vi "220512-VNA RP FLAT.vi"() -> ()   [LabVIEW 2021]
uses:
  Channel parameters.ctl
  Spectrum data.ctl
  vna settings.ctl
  Resonnance detection.ctl
  <vilib>/Analysis/baseanly.llb/Mean (DBL).vi
  <vilib>/Utility/file.llb/Write Delimited Spreadsheet (DBL).vi
  <vilib>/regexp/Match Regular Expression.xnode
  <vilib>/Analysis/NI_AALBase.lvlib
panel:
  in  "Enable optical switch":bool
  in  "RP VNA SETTING":T1={"F start"=200000, "F stop"=2000500, "Sweep size"=1000, "Decimation"=5000, "F_corr"=0, "Ph_OUT1"=0, "Ph_OUT2"=0, "OUT_Lvl1"=32700, "OUT_Lvl2"=32700, "GPIO"=0}
  in  "Amplitude(1V)":dbl=0.3 format="%#_13g"
  out "RP CONNECT":bool
  in  "VOA Calibration cluster":cluster{"PUMP":dbl[], "PROBE":dbl[]}
  out "TRACK DATA REL NO SMOOTHING":dbl[][](array[numeric])
  out "TRACK DATA ABS NO SMOOTHING":dbl[][](array[numeric])
  in  "BTN SAVE TRACK":bool
  in  "BTN STOP TRACK":bool
  out "TRACK REPOSITERY":path
  out "TRACK DATA REL":dbl[][](array[numeric])
  out "TRACK DATA ABS":dbl[][](array[numeric])
  out "Track File List":path[](array[path])
  out "Track Repositery List":path[](array[path])
  out "CHANNEL CHOSEN":i32
  in  "TRACK-STOP":bool
  out "STATUS":string="STOP"
  out "track data":dbl[](array[numeric])=[495490.5081042979, 495481.56129759253, 495478.2328599854, 495479.84884744807, 495476.377462383, 495478.7819904735]
  out "MAIN TAB":T2(tab)
  in  "AVG Nb":i32=1 min=0 max=100 step=1
  in  "BTN AVG ENABLE":bool caption="AVERAGING"
  out "ACQ Indicator":bool
  in  "PUMP":dbl(slide)=100.0 min=0.0 max=100.0 step=0.1 scale=0.0..100.0
  in  "PROBE":dbl(slide)=100.0 min=0.0 max=100.0 step=0.1 scale=0.0..100.0
  in  "BTN RESET VNA":bool
  in  "SPAN":dbl=1900.0 format="%#5.1f"
  in  "STOP":dbl=2000.0 min=0.0 max=3000.0 format="%#5.1f"
  in  "CENTER":dbl=1050.0 format="%#5.1f"
  in  "BTN AF VNA":bool
  out "MAGNITUDE/PHASE":cluster{cluster{dbl, dbl}[]}[](graph)
  in  "CHANNEL CHOICE VNA":T3(radio)
  in  "BTN Center to max":bool
  in  "BTN ZOOM-":bool
  in  "BTN ZOOM+":bool
  in  "START":dbl=200.0 format="%#5.1f"
  out "SPACING":dbl=1900.0 min=0.0 max=100.0 step=0.5 format="%#5.1f"
  in  "Points N°":i32=1000 min=600 max=5000 step=1 format="%#4.4g"
  in  "BTN LOOP VNA":bool
  in  "BTN RUN VNA":bool
  in  "BTN SAVE VNA":bool
  in  "BTN FIT DISPLAY":bool caption="FIT DISPLAY"
  in  "BTN AUTOSCALE":bool=TRUE caption="AUTOSCALE"
  in  "BTN DISPLAY TYPE":bool caption="DISPLAY"
  in  "BTN VIEW PERSISTANCE":bool
  in  "BTN MAG/VEL":bool caption="DISPLAY"
  out "AVG Curr":i32=1 min=0 max=100 step=1
  in  "Hide/Show track data channel":bool[](array[boolean])
  in  "BTN AUTOSAVE RAW DATA":bool=TRUE
  in  "COMMENTS":string
  in  "ASSAY NAME":string
  in  "DELAY AFTER SWITCH (s)":i32
  in  "N°POINTS TO DISPLAY":i32=200
  in  "DISPLAY OPTION":u16(ring) items=["Absolute frequency", "Relative frequency (ppm)"]
  in  "DELAY BETWEEN TRIG (s)":i32
  in  "AVERAGE/POINT":dbl=1.0
  out "LIVE TRACK":dbl[][](graph)
  out "CHANNELS IND TRACK":T3(radio)
  in  "BTN RUN TRACK":bool
  in  "TEMPORAL SMOOTHING":i32=15
  in  "BTN NEW TRACK":bool
  in  "BTN PAUSE TRACK":bool
  in  "CHANNELS PARAMETERS":T4[](array[typedef])=[{"START 2"=200.0, "STOP 2"=2000.5, "CENTER 2"=1050.0, "SPAN 2"=1800.0, "CHANNEL TRACK ?"=FALSE, "PUMP"=100.0, "PROBE"=100.0, "Points N° 2"=1000, "SPACING 2"=100.0, "AVG"=0, "AVG ENABLE"=FALSE}, {"START 2"=200.0, "STOP 2"=2000.0, "CENTER 2"=1100.0, "SPAN 2"=1800.0, "CHANNEL TRACK ?"=FALSE, "PUMP"=100.0, "PROBE"=100.0, "Points N° 2"=1000, "SPACING 2"=1800.0, "AVG"=0, "AVG ENABLE"=FALSE}, {"START 2"=200.0, "STOP 2"=2000.0, "CENTER 2"=1100.0, "SPAN 2"=1800.0, "CHANNEL TRACK ?"=FALSE, "PUMP"=100.0, "PROBE"=100.0, "Points N° 2"=1000, "SPACING 2"=1800.0, "AVG"=0, "AVG ENABLE"=FALSE}, {"START 2"=200.0, "STOP 2"=2000.0, "CENTER 2"=1100.0, "SPAN 2"=1800.0, "CHANNEL TRACK ?"=FALSE, "PUMP"=100.0, "PROBE"=100.0, "Points N° 2"=1000, "SPACING 2"=1800.0, "AVG"=0, "AVG ENABLE"=FALSE}, {"START 2"=200.0, "STOP 2"=2000.0, "CENTER 2"=1100.0, "SPAN 2"=1800.0, "CHANNEL TRACK ?"=FALSE, "PUMP"=100.0, "PROBE"=100.0, "Points N° 2"=1000, "SPACING 2"=1800.0, "AVG"=0, "AVG ENABLE"=FALSE}, {"START 2"=200.0, "STOP 2"=2000.0, "CENTER 2"=1100.0, "SPAN 2"=1800.0, "CHANNEL TRACK ?"=FALSE, "PUMP"=100.0, "PROBE"=100.0, "Points N° 2"=1000, "SPACING 2"=1800.0, "AVG"=0, "AVG ENABLE"=FALSE}, {"START 2"=200.0, "STOP 2"=2000.0, "CENTER 2"=1100.0, "SPAN 2"=1800.0, "CHANNEL TRACK ?"=FALSE, "PUMP"=100.0, "PROBE"=100.0, "Points N° 2"=1000, "SPACING 2"=1800.0, "AVG"=0, "AVG ENABLE"=FALSE}, {"START 2"=200.0, "STOP 2"=2000.0, "CENTER 2"=1100.0, "SPAN 2"=1800.0, "CHANNEL TRACK ?"=FALSE, "PUMP"=100.0, "PROBE"=100.0, "Points N° 2"=1000, "SPACING 2"=1800.0, "AVG"=0, "AVG ENABLE"=FALSE}, {"START 2"=200.0, "STOP 2"=2000.0, "CENTER 2"=1100.0, "SPAN 2"=1800.0, "CHANNEL TRACK ?"=FALSE, "PUMP"=100.0, "PROBE"=100.0, "Points N° 2"=1000, "SPACING 2"=1800.0, "AVG"=0, "AVG ENABLE"=FALSE}, {"START 2"=200.0, "STOP 2"=2000.0, "CENTER 2"=1100.0, "SPAN 2"=1800.0, "CHANNEL TRACK ?"=FALSE, "PUMP"=100.0, "PROBE"=100.0, "Points N° 2"=1000, "SPACING 2"=1800.0, "AVG"=0, "AVG ENABLE"=FALSE}, {"START 2"=200.0, "STOP 2"=2000.0, "CENTER 2"=1100.0, "SPAN 2"=1800.0, "CHANNEL TRACK ?"=FALSE, "PUMP"=100.0, "PROBE"=100.0, "Points N° 2"=1000, "SPACING 2"=1800.0, "AVG"=0, "AVG ENABLE"=FALSE}, {"START 2"=200.0, "STOP 2"=2000.0, "CENTER 2"=1100.0, "SPAN 2"=1800.0, "CHANNEL TRACK ?"=FALSE, "PUMP"=100.0, "PROBE"=100.0, "Points N° 2"=1000, "SPACING 2"=1800.0, "AVG"=0, "AVG ENABLE"=FALSE}, {"START 2"=200.0, "STOP 2"=2000.0, "CENTER 2"=1100.0, "SPAN 2"=1800.0, "CHANNEL TRACK ?"=FALSE, "PUMP"=100.0, "PROBE"=100.0, "Points N° 2"=1000, "SPACING 2"=1800.0, "AVG"=0, "AVG ENABLE"=FALSE}, {"START 2"=200.0, "STOP 2"=2000.0, "CENTER 2"=1100.0, "SPAN 2"=1800.0, "CHANNEL TRACK ?"=FALSE, "PUMP"=100.0, "PROBE"=100.0, "Points N° 2"=1000, "SPACING 2"=1800.0, "AVG"=0, "AVG ENABLE"=FALSE}, {"START 2"=200.0, "STOP 2"=2000.0, "CENTER 2"=1100.0, "SPAN 2"=1800.0, "CHANNEL TRACK ?"=FALSE, "PUMP"=100.0, "PROBE"=100.0, "Points N° 2"=1000, "SPACING 2"=1800.0, "AVG"=0, "AVG ENABLE"=FALSE}, {"START 2"=200.0, "STOP 2"=2000.0, "CENTER 2"=1100.0, "SPAN 2"=1800.0, "CHANNEL TRACK ?"=FALSE, "PUMP"=100.0, "PROBE"=100.0, "Points N° 2"=1000, "SPACING 2"=1800.0, "AVG"=0, "AVG ENABLE"=FALSE}] {"AVG" min=0 max=100 step=1; "SPACING 2" min=0.0 max=100.0 step=0.5; "Points N° 2" min=0 max=100 step=1; "PROBE" min=0.0 max=100.0 step=0.5; "PUMP" min=0.0 max=100.0 step=0.5}
  out "CHANNEL IND SETTINGS":T5(radio)
  in  "RESONNANCE DETECTION":T6={"METHOD"=0, "Parabolic fit"={"Span type"=0, "Fit span"=100.0}} {"Parabolic fit"."Span type" items=["Points N°", "Frequency (Hz)", "Span %"]; "METHOD" items=["Maximum amplitude", "Max on parabolic fit"]}
  in  "TRACK DATA PARAMETERS":cluster{"MAIN FOLDER":path}={"MAIN FOLDER"=path "C:/SensWay Data"}
  in  "SPECTRUM POST PROCESSING PARAMETERS":cluster{"N° SMOOTHING POINTS":i32}={"N° SMOOTHING POINTS"=50}
  in  "AUTOFOCUS PARAMETERS":cluster{"ITERATIONS":i32}={"ITERATIONS"=5}
  in  "CHANNELS":T7
  in  "NETWORK PARAMETERS":T8={"RP-IP 1"="192.168.0.3", "RP-IP 2"="192.168.0.4", "RP-MAC 1"="", "RP-MAC 2"=""}
  in  "DARK SUB ?":bool
  in  "VNA DATA CLUSTER":T9 {"Time Stamp Indicator - Long" format="%<%.0X %x>T"}
  in  "TRACK DATA CLUSTER":cluster{"CHANNEL":dbl, "KPI 1 TRACK":ext[]}
  out "LOOP ACT":bool
  out "RAW Freq table":dbl[](array[numeric])=[200000.0, 201802.3023023023, 203604.6046046046, 205406.9069069069, 207209.20920920922, 209011.51151151152, 210813.81381381382, 212616.1161161161, 214418.4184184184, 216220.7207207207, 218023.02302302304, 219825.32532532534, 221627.62762762763, 223429.92992992993, 225232.23223223223, 227034.53453453453, 228836.83683683682, 230639.13913913915, 232441.44144144145, 234243.74374374375, 236046.04604604605, 237848.34834834834, 239650.65065065064, 241452.95295295294, 243255.25525525527, 245057.55755755756, 246859.85985985986, 248662.16216216216, 250464.46446446446, 252266.76676676676, 254069.06906906905, 255871.37137137138, 257673.67367367368, 259475.97597597598, 261278.27827827827, 263080.5805805806, 264882.8828828829, 266685.18518518517, 268487.4874874875, 270289.7897897898, 272092.0920920921, 273894.39439439436, 275696.6966966967, 277498.998998999, 279301.3013013013, 281103.6036036036, 282905.9059059059, 284708.2082082082, 286510.51051051053, 288312.8128128128, 290115.1151151151, 291917.4174174174, 293719.7197197197, 295522.02202202205, 297324.3243243243, 299126.6266266266, 300928.9289289289, 302731.23123123124, 304533.5335335335, 306335.83583583584, 308138.1381381381, 309940.44044044043, 311742.74274274276, 313545.04504504503, 315347.34734734736, 317149.6496496496, 318951.95195195195, 320754.2542542543, 322556.55655655655, 324358.8588588588, 326161.16116116114, 327963.4634634635, 329765.76576576574, 331568.06806806807, 333370.37037037034, 335172.67267267266, 336974.974974975, 338777.27727727726, 340579.5795795796, 342381.88188188185, 344184.1841841842, 345986.4864864865, 347788.7887887888, 349591.09109109105, 351393.3933933934, 353195.6956956957, 354997.997997998, 356800.3003003003, 358602.60260260256, 360404.9049049049, 362207.2072072072, 364009.50950950955, 365811.8118118118, 367614.1141141141, 369416.4164164164, 371218.71871871874, 373021.021021021, 374823.3233233233, 376625.6256256256, 378427.9279279279, 380230.23023023026, 382032.5325325325, 383834.8348348348, 385637.1371371371, 387439.43943943945, 389241.7417417418, 391044.04404404404, 392846.3463463463, 394648.64864864864, 396450.95095095097, 398253.25325325324, 400055.5555555555, 401857.85785785783, 403660.16016016016, 405462.4624624625, 407264.76476476475, 409067.067067067, 410869.36936936935, 412671.6716716717, 414473.973973974, 416276.2762762763, 418078.57857857854, 419880.88088088087, 421683.1831831832, 423485.48548548546, 425287.7877877878, 427090.09009009006, 428892.3923923924, 430694.6946946947, 432496.996996997, 434299.29929929925, 436101.6016016016, 437903.9039039039, 439706.20620620623, 441508.5085085085, 443310.81081081077, 445113.1131131131, 446915.4154154154, 448717.7177177177, 450520.02002002, 452322.3223223223, 454124.6246246246, 455926.92692692694, 457729.2292292292, 459531.5315315315, 461333.8338338338, 463136.13613613613, 464938.4384384384, 466740.74074074073, 468543.04304304306, 470345.3453453453, 472147.64764764765, 473949.9499499499, 475752.25225225225, 477554.5545545545, 479356.85685685684, 481159.1591591592, 482961.46146146144, 484763.76376376377, 486566.06606606604, 488368.36836836836, 490170.67067067063, 491972.97297297296, 493775.2752752753, 495577.57757757755, 497379.8798798799, 499182.18218218215, 500984.4844844845, 502786.78678678675, 504589.0890890891, 506391.3913913914, 508193.69369369367, 509995.995995996, 511798.29829829826, 513600.6006006006, 515402.90290290286, 517205.2052052052, 519007.5075075075, 520809.8098098098, 522612.1121121121, 524414.4144144144, 526216.7167167168, 528019.0190190191, 529821.3213213213, 531623.6236236236, 533425.9259259258, 535228.2282282282, 537030.5305305305, 538832.8328328328, 540635.1351351351, 542437.4374374375, 544239.7397397398, 546042.042042042, 547844.3443443443, 549646.6466466465, 551448.9489489489, 553251.2512512512, 555053.5535535535, 556855.8558558559, 558658.1581581582, 560460.4604604605, 562262.7627627627, 564065.065065065, 565867.3673673674, 567669.6696696696, 569471.9719719719, 571274.2742742742, 573076.5765765766, 574878.8788788789, 576681.1811811812, 578483.4834834835, 580285.7857857858, 582088.0880880881, 583890.3903903903, 585692.6926926926, 587494.994994995, 589297.2972972973, 591099.5995995996, 592901.9019019019, 594704.2042042043, 596506.5065065065, 598308.8088088088, 600111.111111111, 601913.4134134133, 603715.7157157157, 605518.018018018, 607320.3203203203, 609122.6226226226, 610924.924924925, 612727.2272272272, 614529.5295295295, 616331.8318318318, 618134.134134134, 619936.4364364364, 621738.7387387387, 623541.041041041, 625343.3433433434, 627145.6456456457, 628947.947947948, 630750.2502502502, 632552.5525525525, 634354.8548548548, 636157.1571571571, 637959.4594594594, 639761.7617617617, 641564.0640640641, 643366.3663663664, 645168.6686686687, 646970.9709709709, 648773.2732732733, 650575.5755755756, 652377.8778778778, 654180.1801801801, 655982.4824824824, 657784.7847847848, 659587.0870870871, 661389.3893893894, 663191.6916916918, 664993.993993994, 666796.2962962963, 668598.5985985985, 670400.9009009008, 672203.2032032032, 674005.5055055055, 675807.8078078078, 677610.1101101101, 679412.4124124125, 681214.7147147147, 683017.017017017, 684819.3193193192, 686621.6216216215, 688423.9239239239, 690226.2262262262, 692028.5285285285, 693830.8308308308, 695633.1331331332, 697435.4354354354, 699237.7377377377, 701040.04004004, 702842.3423423423, 704644.6446446446, 706446.9469469469, 708249.2492492492, 710051.5515515516, 711853.8538538539, 713656.1561561562, 715458.4584584584, 717260.7607607607, 719063.063063063, 720865.3653653653, 722667.6676676676, 724469.9699699699, 726272.2722722723, 728074.5745745746, 729876.8768768768, 731679.1791791791, 733481.4814814815, 735283.7837837838, 737086.0860860861, 738888.3883883883, 740690.6906906907, 742492.992992993, 744295.2952952953, 746097.5975975975, 747899.8998998998, 749702.2022022022, 751504.5045045045, 753306.8068068068, 755109.109109109, 756911.4114114114, 758713.7137137137, 760516.016016016, 762318.3183183183, 764120.6206206206, 765922.9229229229, 767725.2252252252, 769527.5275275275, 771329.8298298299, 773132.1321321321, 774934.4344344344, 776736.7367367367, 778539.039039039, 780341.3413413413, 782143.6436436436, 783945.9459459459, 785748.2482482482, 787550.5505505506, 789352.8528528528, 791155.1551551551, 792957.4574574574, 794759.7597597598, 796562.0620620621, 798364.3643643643, 800166.6666666666, 801968.968968969, 803771.2712712713, 805573.5735735735, 807375.8758758758, 809178.1781781781, 810980.4804804805, 812782.7827827828, 814585.085085085, 816387.3873873873, 818189.6896896897, 819991.991991992, 821794.2942942943, 823596.5965965965, 825398.8988988989, 827201.2012012012, 829003.5035035035, 830805.8058058057, 832608.108108108, 834410.4104104104, 836212.7127127127, 838015.015015015, 839817.3173173172, 841619.6196196196, 843421.9219219219, 845224.2242242242, 847026.5265265265, 848828.8288288288, 850631.1311311311, 852433.4334334334, 854235.7357357357, 856038.0380380381, 857840.3403403403, 859642.6426426426, 861444.9449449449, 863247.2472472473, 865049.5495495495, 866851.8518518518, 868654.1541541541, 870456.4564564564, 872258.7587587588, 874061.061061061, 875863.3633633633, 877665.6656656656, 879467.967967968, 881270.2702702703, 883072.5725725725, 884874.8748748748, 886677.1771771772, 888479.4794794795, 890281.7817817817, 892084.084084084, 893886.3863863864, 895688.6886886887, 897490.990990991, 899293.2932932932, 901095.5955955955, 902897.8978978979, 904700.2002002002, 906502.5025025025, 908304.8048048047, 910107.1071071071, 911909.4094094094, 913711.7117117117, 915514.0140140139, 917316.3163163163, 919118.6186186186, 920920.9209209209, 922723.2232232232, 924525.5255255254, 926327.8278278278, 928130.1301301301, 929932.4324324324, 931734.7347347348, 933537.037037037, 935339.3393393393, 937141.6416416416, 938943.943943944, 940746.2462462463, 942548.5485485485, 944350.8508508508, 946153.1531531531, 947955.4554554555, 949757.7577577577, 951560.06006006, 953362.3623623623, 955164.6646646647, 956966.966966967, 958769.2692692692, 960571.5715715715, 962373.8738738738, 964176.1761761762, 965978.4784784785, 967780.7807807807, 969583.083083083, 971385.3853853854, 973187.6876876877, 974989.9899899899, 976792.2922922922, 978594.5945945946, 980396.8968968969, 982199.1991991992, 984001.5015015014, 985803.8038038037, 987606.1061061061, 989408.4084084084, 991210.7107107107, 993013.0130130129, 994815.3153153153, 996617.6176176176, 998419.9199199199, 1000222.2222222221, 1002024.5245245245, 1003826.8268268268, 1005629.1291291291, 1007431.4314314314, 1009233.7337337337, 1011036.036036036, 1012838.3383383383, 1014640.6406406406, 1016442.942942943, 1018245.2452452452, 1020047.5475475475, 1021849.8498498498, 1023652.1521521521, 1025454.4544544544, 1027256.7567567567, 1029059.059059059, 1030861.3613613613, 1032663.6636636637, 1034465.9659659659, 1036268.2682682682, 1038070.5705705705, 1039872.8728728729, 1041675.1751751752, 1043477.4774774774, 1045279.7797797797, 1047082.082082082, 1048884.3843843844, 1050686.6866866867, 1052488.988988989, 1054291.2912912914, 1056093.5935935937, 1057895.895895896, 1059698.198198198, 1061500.5005005004, 1063302.8028028028, 1065105.105105105, 1066907.4074074074, 1068709.7097097095, 1070512.0120120118, 1072314.3143143142, 1074116.6166166165, 1075918.9189189188, 1077721.2212212211, 1079523.5235235235, 1081325.8258258258, 1083128.1281281281, 1084930.4304304305, 1086732.7327327328, 1088535.035035035, 1090337.3373373374, 1092139.6396396398, 1093941.9419419419, 1095744.2442442442, 1097546.5465465465, 1099348.8488488488, 1101151.1511511512, 1102953.4534534533, 1104755.7557557556, 1106558.058058058, 1108360.3603603602, 1110162.6626626626, 1111964.964964965, 1113767.2672672672, 1115569.5695695695, 1117371.8718718719, 1119174.1741741742, 1120976.4764764765, 1122778.7787787789, 1124581.0810810812, 1126383.3833833835, 1128185.6856856856, 1129987.987987988, 1131790.2902902903, 1133592.5925925926, 1135394.894894895, 1137197.197197197, 1138999.4994994993, 1140801.8018018017, 1142604.104104104, 1144406.4064064063, 1146208.7087087086, 1148011.011011011, 1149813.3133133133, 1151615.6156156156, 1153417.917917918, 1155220.2202202203, 1157022.5225225226, 1158824.824824825, 1160627.1271271273, 1162429.4294294294, 1164231.7317317317, 1166034.034034034, 1167836.3363363363, 1169638.6386386384, 1171440.9409409408, 1173243.243243243, 1175045.5455455454, 1176847.8478478477, 1178650.15015015, 1180452.4524524524, 1182254.7547547547, 1184057.057057057, 1185859.3593593594, 1187661.6616616617, 1189463.963963964, 1191266.2662662663, 1193068.5685685687, 1194870.8708708708, 1196673.173173173, 1198475.4754754754, 1200277.7777777778, 1202080.08008008, 1203882.3823823822, 1205684.6846846845, 1207486.9869869868, 1209289.2892892892, 1211091.5915915915, 1212893.8938938938, 1214696.1961961961, 1216498.4984984985, 1218300.8008008008, 1220103.103103103, 1221905.4054054054, 1223707.7077077078, 1225510.01001001, 1227312.3123123124, 1229114.6146146145, 1230916.9169169168, 1232719.2192192192, 1234521.5215215215, 1236323.8238238238, 1238126.126126126, 1239928.4284284282, 1241730.7307307306, 1243533.033033033, 1245335.3353353352, 1247137.6376376376, 1248939.9399399399, 1250742.2422422422, 1252544.5445445445, 1254346.8468468469, 1256149.1491491492, 1257951.4514514515, 1259753.7537537536, 1261556.056056056, 1263358.3583583583, 1265160.6606606606, 1266962.962962963, 1268765.2652652652, 1270567.5675675676, 1272369.86986987, 1274172.1721721722, 1275974.4744744743, 1277776.7767767766, 1279579.079079079, 1281381.3813813813, 1283183.6836836836, 1284985.985985986, 1286788.2882882883, 1288590.5905905906, 1290392.892892893, 1292195.195195195, 1293997.4974974974, 1295799.7997997997, 1297602.102102102, 1299404.4044044043, 1301206.7067067067, 1303009.009009009, 1304811.3113113113, 1306613.6136136136, 1308415.915915916, 1310218.218218218, 1312020.5205205204, 1313822.8228228227, 1315625.125125125, 1317427.4274274274, 1319229.7297297297, 1321032.032032032, 1322834.3343343344, 1324636.6366366367, 1326438.9389389388, 1328241.241241241, 1330043.5435435434, 1331845.8458458458, 1333648.148148148, 1335450.4504504504, 1337252.7527527527, 1339055.055055055, 1340857.3573573574, 1342659.6596596597, 1344461.9619619618, 1346264.2642642641, 1348066.5665665665, 1349868.8688688688, 1351671.1711711711, 1353473.4734734735, 1355275.7757757758, 1357078.078078078, 1358880.3803803804, 1360682.6826826825, 1362484.9849849849, 1364287.2872872872, 1366089.5895895895, 1367891.8918918918, 1369694.1941941942, 1371496.4964964965, 1373298.7987987988, 1375101.1011011011, 1376903.4034034032, 1378705.7057057056, 1380508.008008008, 1382310.3103103102, 1384112.6126126125, 1385914.9149149149, 1387717.2172172172, 1389519.5195195195, 1391321.8218218219, 1393124.1241241242, 1394926.4264264263, 1396728.7287287286, 1398531.031031031, 1400333.3333333333, 1402135.6356356356, 1403937.937937938, 1405740.2402402402, 1407542.5425425426, 1409344.844844845, 1411147.147147147, 1412949.4494494493, 1414751.7517517516, 1416554.054054054, 1418356.3563563563, 1420158.6586586586, 1421960.960960961, 1423763.2632632633, 1425565.5655655656, 1427367.867867868, 1429170.17017017, 1430972.4724724723, 1432774.7747747747, 1434577.077077077, 1436379.3793793793, 1438181.6816816817, 1439983.983983984, 1441786.2862862863, 1443588.5885885886, 1445390.8908908907, 1447193.193193193, 1448995.4954954954, 1450797.7977977977, 1452600.1001001, 1454402.4024024024, 1456204.7047047047, 1458007.007007007, 1459809.3093093093, 1461611.6116116114, 1463413.9139139138, 1465216.216216216, 1467018.5185185184, 1468820.8208208208, 1470623.123123123, 1472425.4254254254, 1474227.7277277277, 1476030.03003003, 1477832.3323323324, 1479634.6346346345, 1481436.9369369368, 1483239.2392392391, 1485041.5415415415, 1486843.8438438438, 1488646.146146146, 1490448.4484484484, 1492250.7507507508, 1494053.053053053, 1495855.3553553552, 1497657.6576576575, 1499459.9599599598, 1501262.2622622622, 1503064.5645645645, 1504866.8668668668, 1506669.1691691692, 1508471.4714714715, 1510273.7737737738, 1512076.0760760761, 1513878.3783783782, 1515680.6806806806, 1517482.9829829829, 1519285.2852852852, 1521087.5875875875, 1522889.8898898899, 1524692.1921921922, 1526494.4944944945, 1528296.7967967968, 1530099.099099099, 1531901.4014014013, 1533703.7037037036, 1535506.006006006, 1537308.3083083082, 1539110.6106106106, 1540912.912912913, 1542715.2152152152, 1544517.5175175176, 1546319.8198198196, 1548122.122122122, 1549924.4244244243, 1551726.7267267266, 1553529.029029029, 1555331.3313313313, 1557133.6336336336, 1558935.935935936, 1560738.2382382383, 1562540.5405405406, 1564342.8428428427, 1566145.145145145, 1567947.4474474473, 1569749.7497497497, 1571552.052052052, 1573354.3543543543, 1575156.6566566566, 1576958.958958959, 1578761.2612612613, 1580563.5635635634, 1582365.8658658657, 1584168.168168168, 1585970.4704704704, 1587772.7727727727, 1589575.075075075, 1591377.3773773774, 1593179.6796796797, 1594981.981981982, 1596784.2842842843, 1598586.5865865864, 1600388.8888888888, 1602191.191191191, 1603993.4934934934, 1605795.7957957957, 1607598.098098098, 1609400.4004004004, 1611202.7027027027, 1613005.005005005, 1614807.3073073071, 1616609.6096096095, 1618411.9119119118, 1620214.2142142141, 1622016.5165165165, 1623818.8188188188, 1625621.121121121, 1627423.4234234234, 1629225.7257257258, 1631028.0280280279, 1632830.3303303302, 1634632.6326326325, 1636434.9349349348, 1638237.2372372372, 1640039.5395395395, 1641841.8418418418, 1643644.1441441441, 1645446.4464464465, 1647248.7487487488, 1649051.051051051, 1650853.3533533532, 1652655.6556556555, 1654457.9579579579, 1656260.2602602602, 1658062.5625625625, 1659864.8648648649, 1661667.1671671672, 1663469.4694694695, 1665271.7717717716, 1667074.074074074, 1668876.3763763763, 1670678.6786786786, 1672480.980980981, 1674283.2832832832, 1676085.5855855856, 1677887.887887888, 1679690.1901901902, 1681492.4924924925, 1683294.7947947946, 1685097.097097097, 1686899.3993993993, 1688701.7017017016, 1690504.004004004, 1692306.3063063063, 1694108.6086086086, 1695910.910910911, 1697713.2132132133, 1699515.5155155153, 1701317.8178178177, 1703120.12012012, 1704922.4224224223, 1706724.7247247247, 1708527.027027027, 1710329.3293293293, 1712131.6316316316, 1713933.933933934, 1715736.236236236, 1717538.5385385384, 1719340.8408408407, 1721143.143143143, 1722945.4454454454, 1724747.7477477477, 1726550.05005005, 1728352.3523523523, 1730154.6546546547, 1731956.956956957, 1733759.259259259, 1735561.5615615614, 1737363.8638638637, 1739166.166166166, 1740968.4684684684, 1742770.7707707707, 1744573.073073073, 1746375.3753753754, 1748177.6776776777, 1749979.9799799798, 1751782.2822822821, 1753584.5845845845, 1755386.8868868868, 1757189.189189189, 1758991.4914914914, 1760793.7937937938, 1762596.096096096, 1764398.3983983984, 1766200.7007007005, 1768003.0030030028, 1769805.3053053052, 1771607.6076076075, 1773409.9099099098, 1775212.2122122122, 1777014.5145145145, 1778816.8168168168, 1780619.1191191191, 1782421.4214214215, 1784223.7237237236, 1786026.0260260259, 1787828.3283283282, 1789630.6306306305, 1791432.9329329329, 1793235.2352352352, 1795037.5375375375, 1796839.8398398398, 1798642.1421421422, 1800444.4444444443, 1802246.7467467466, 1804049.049049049, 1805851.3513513512, 1807653.6536536536, 1809455.955955956, 1811258.2582582582, 1813060.5605605606, 1814862.8628628629, 1816665.1651651652, 1818467.4674674673, 1820269.7697697696, 1822072.072072072, 1823874.3743743743, 1825676.6766766766, 1827478.978978979, 1829281.2812812813, 1831083.5835835836, 1832885.885885886, 1834688.188188188, 1836490.4904904903, 1838292.7927927927, 1840095.095095095, 1841897.3973973973, 1843699.6996996996, 1845502.002002002, 1847304.3043043043, 1849106.6066066066, 1850908.9089089087, 1852711.211211211, 1854513.5135135134, 1856315.8158158157, 1858118.118118118, 1859920.4204204204, 1861722.7227227227, 1863525.025025025, 1865327.3273273273, 1867129.6296296297, 1868931.9319319318, 1870734.234234234, 1872536.5365365364, 1874338.8388388387, 1876141.141141141, 1877943.4434434434, 1879745.7457457457, 1881548.048048048, 1883350.3503503504, 1885152.6526526525, 1886954.9549549548, 1888757.2572572571, 1890559.5595595594, 1892361.8618618618, 1894164.164164164, 1895966.4664664664, 1897768.7687687688, 1899571.071071071, 1901373.3733733734, 1903175.6756756755, 1904977.9779779778, 1906780.2802802802, 1908582.5825825825, 1910384.8848848848, 1912187.1871871871, 1913989.4894894895, 1915791.7917917918, 1917594.0940940941, 1919396.3963963962, 1921198.6986986985, 1923001.0010010009, 1924803.3033033032, 1926605.6056056055, 1928407.9079079079, 1930210.2102102102, 1932012.5125125125, 1933814.8148148148, 1935617.117117117, 1937419.4194194193, 1939221.7217217216, 1941024.024024024, 1942826.3263263262, 1944628.6286286286, 1946430.930930931, 1948233.2332332332, 1950035.5355355355, 1951837.8378378379, 1953640.14014014, 1955442.4424424423, 1957244.7447447446, 1959047.047047047, 1960849.3493493493, 1962651.6516516516, 1964453.953953954, 1966256.2562562563, 1968058.5585585586, 1969860.8608608607, 1971663.163163163, 1973465.4654654653, 1975267.7677677677, 1977070.07007007, 1978872.3723723723, 1980674.6746746746, 1982476.976976977, 1984279.2792792793, 1986081.5815815816, 1987883.8838838837, 1989686.186186186, 1991488.4884884884, 1993290.7907907907, 1995093.093093093, 1996895.3953953953, 1998697.6976976977, 2000500.0]
  in  "ENABLE INTERNAL MODULATION":bool=TRUE
  in  "VNA DATA CLUSTER TBL":T9[](array[typedef]) {"Time Stamp Indicator - Long" format="%<%.0X %x>T"}
  in  "TRACK DATA CLUSTER TBL":cluster{"CHANNEL":dbl, "KPI 1 TRACK":ext[]}[](array[cluster])=[{"CHANNEL"=0.0, "KPI 1 TRACK"=[]}, {"CHANNEL"=0.0, "KPI 1 TRACK"=[]}, {"CHANNEL"=0.0, "KPI 1 TRACK"=[]}, {"CHANNEL"=0.0, "KPI 1 TRACK"=[]}, {"CHANNEL"=0.0, "KPI 1 TRACK"=[]}, {"CHANNEL"=0.0, "KPI 1 TRACK"=[]}, {"CHANNEL"=0.0, "KPI 1 TRACK"=[]}, {"CHANNEL"=0.0, "KPI 1 TRACK"=[]}, {"CHANNEL"=0.0, "KPI 1 TRACK"=[]}, {"CHANNEL"=0.0, "KPI 1 TRACK"=[]}, {"CHANNEL"=0.0, "KPI 1 TRACK"=[]}, {"CHANNEL"=0.0, "KPI 1 TRACK"=[]}, {"CHANNEL"=0.0, "KPI 1 TRACK"=[]}, {"CHANNEL"=0.0, "KPI 1 TRACK"=[]}, {"CHANNEL"=0.0, "KPI 1 TRACK"=[]}, {"CHANNEL"=0.0, "KPI 1 TRACK"=[]}]
  in  "PERSISTANCE DATA CLUSTER":T9 {"Time Stamp Indicator - Long" format="%<%.0X %x>T"}
  in  "VNA SETTING CLUSTER":T4 {"AVG" min=0 max=100 step=1; "SPACING 2" min=0.0 max=100.0 step=0.5; "Points N° 2" min=0 max=100 step=1; "PROBE" min=0.0 max=100.0 step=0.5; "PUMP" min=0.0 max=100.0 step=0.5}
  out "Information tips":string
  in  "PANEL VNA":bool
  in  "PANEL TRACKING":bool
  in  "BTN STOP":bool
  in  "PANEL GENERAL SETTINGS":bool
  in  "PANEL TRACK SETTINGS":bool
  # "POINTS"
  # "SPACING"
  # "TRACK ?"
  # "START"
  # "STOP"
  # "CENTER"
  # "SPAN"
  # "PROBE"
  # "PUMP"
  # "AVERAGING"
  # "BETA ONLY !!!"
  # "PARAMETERS"
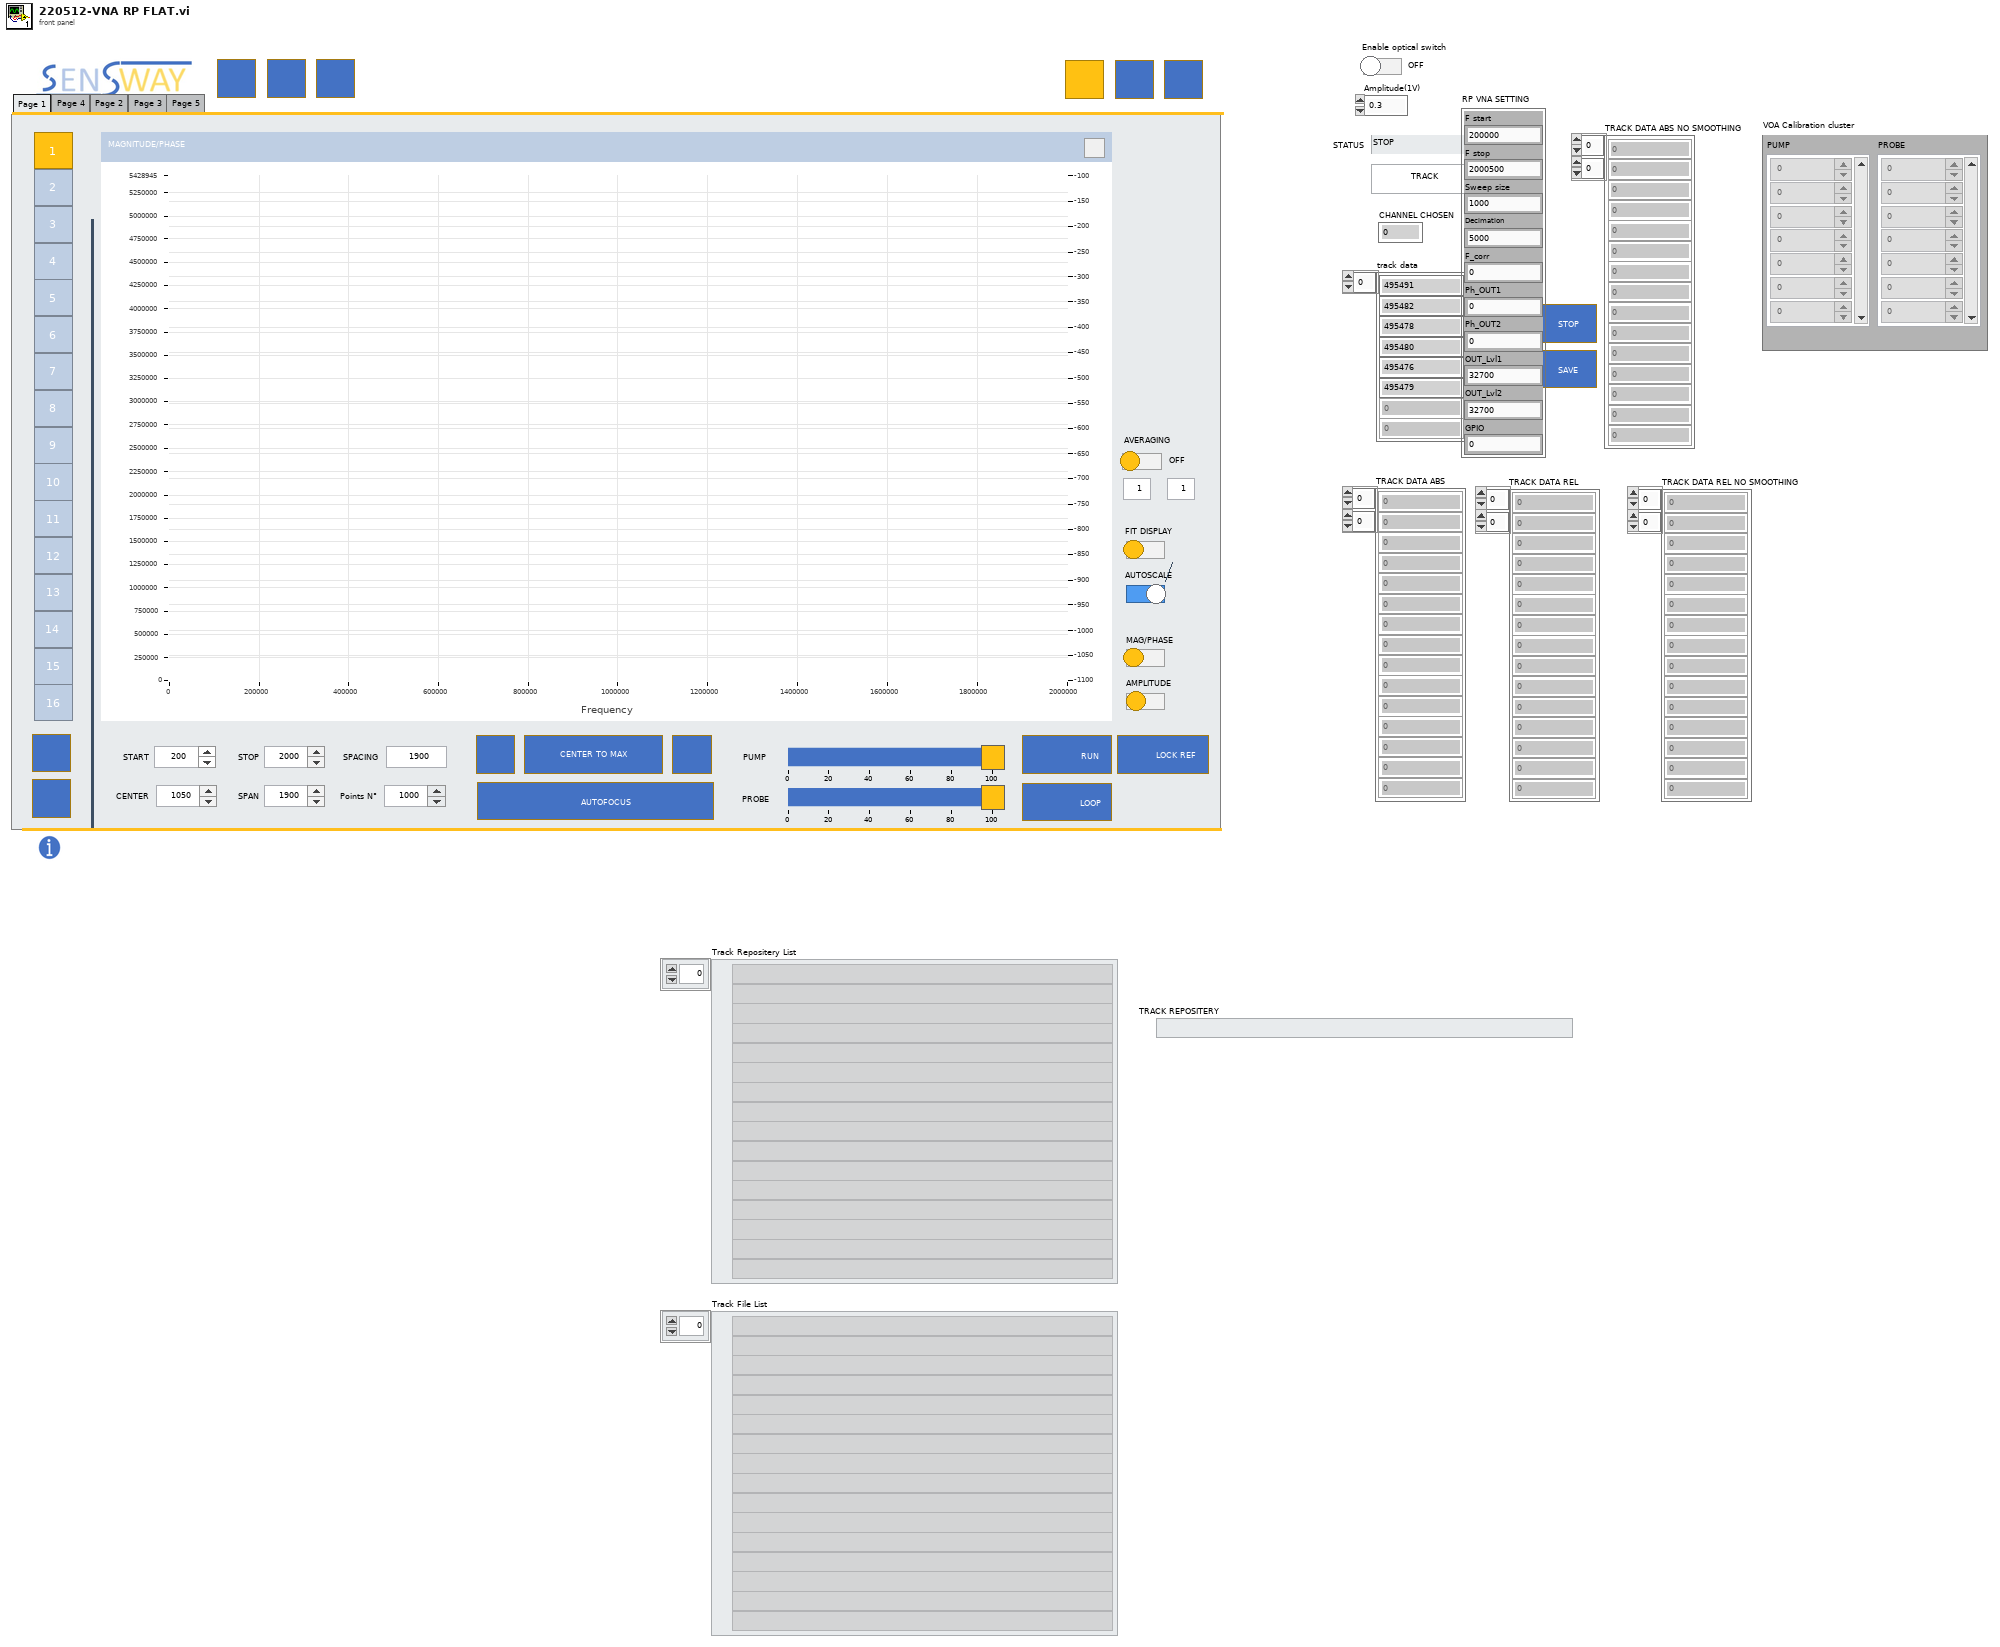
[diagram p1: front panel]
types:
  T1 = typedef "vna settings.ctl" = cluster{"F start":u32, "F stop":u32, "Sweep size":u32, "Decimation":u32, "F_corr":u32, "Ph_OUT1":u32, "Ph_OUT2":u32, "OUT_Lvl1":u32, "OUT_Lvl2":u32, "GPIO":u32}
  T2 = enum32{"Page 1", "Page 4", "Page 2", "Page 3", "Page 5"}
  T3 = enum32{"Button 1", "Button 2", "Button 3", "Sélection radio 4", "Sélection radio 5", "Sélection radio 6", "Sélection radio 7", "Sélection radio 8", "Sélection radio 9", "Sélection radio 10", "Sélection radio 11", "Sélection radio 12", "Sélection radio 13", "Sélection radio 14", "Sélection radio 15", "Sélection radio 16"}
  T4 = typedef "Channel parameters.ctl" = cluster{"START 2":dbl, "STOP 2":dbl, "CENTER 2":dbl, "SPAN 2":dbl, "CHANNEL TRACK ?":bool, "PUMP":dbl, "PROBE":dbl, "Points N° 2":i32, "SPACING 2":dbl, "AVG":i32, "AVG ENABLE":bool}
  T5 = enum32{"No Selection", "Button 1", "Button 2", "Button 3", "Sélection radio 4", "Sélection radio 5", "Sélection radio 6", "Sélection radio 7", "Sélection radio 8", "Sélection radio 9", "Sélection radio 10", "Sélection radio 11", "Sélection radio 12", "Sélection radio 13", "Sélection radio 14", "Sélection radio 15", "Sélection radio 16"}
  T6 = typedef "Resonnance detection.ctl" = cluster{"METHOD":u16, "Parabolic fit":cluster{"Span type":u16, "Fit span":dbl}}
  T7 = cluster{"CHANNEL 1":bool, "CHANNEL 2":bool, "CHANNEL 3":bool, "CHANNEL 4":bool, "CHANNEL 5":bool, "CHANNEL 6":bool, "CHANNEL 7":bool, "CHANNEL 8":bool, "CHANNEL 9":bool, "CHANNEL 10":bool, "CHANNEL 11":bool, "CHANNEL 12":bool, "CHANNEL 13":bool, "CHANNEL 14":bool, "CHANNEL 15":bool, "CHANNEL 16":bool}
  T8 = cluster{"RP-IP 1":string, "RP-IP 2":string, "RP-MAC 1":string, "RP-MAC 2":string}
  T9 = typedef "Spectrum data.ctl" = cluster{"CHANNEL":dbl, "FREQUENCY TABLE":ext[], "MAGNITUDE TABLE":ext[], "PHASE TABLE":ext[], "REAL TABLE":ext[], "IMAGINARY TABLE":ext[], "Time Stamp Indicator - Long":timestamp}
  T10 = enum16{"Freq start", "Freq stop", "Sweep size", "Decimation rate", "Freq corr", "Phase output 1", "Phase output 2", "Output level 1", "Output level 2", "GPIO", "SWEEP START"}
  T11 = enum8{"Enabled", "Disabled", "Disabled and Grayed Out"}
  T12 = cluster{"FREQUENCY":sgl[], "REAL 1":dbl[], "IMAGINARY 1":sgl[], "MAGNITUDE 1":dbl[], "PHASE 1":dbl[], "REAL 2":dbl[], "IMAGINARY 2":sgl[], "MAGNITUDE 2":dbl[], "PHASE 2":dbl[]}
  T13 = cluster{cluster{"Numeric Control":ext, "Numeric Control":ext}[]}[]
  T14 = cluster{"F start":u32, "F stop":u32, "Sweep size":u32, "Decimation":u32, "F_corr":u32, "Ph_OUT1":u32, "Ph_OUT2":u32, "OUT_Lvl1":u32, "OUT_Lvl2":u32, "GPIO":u32}
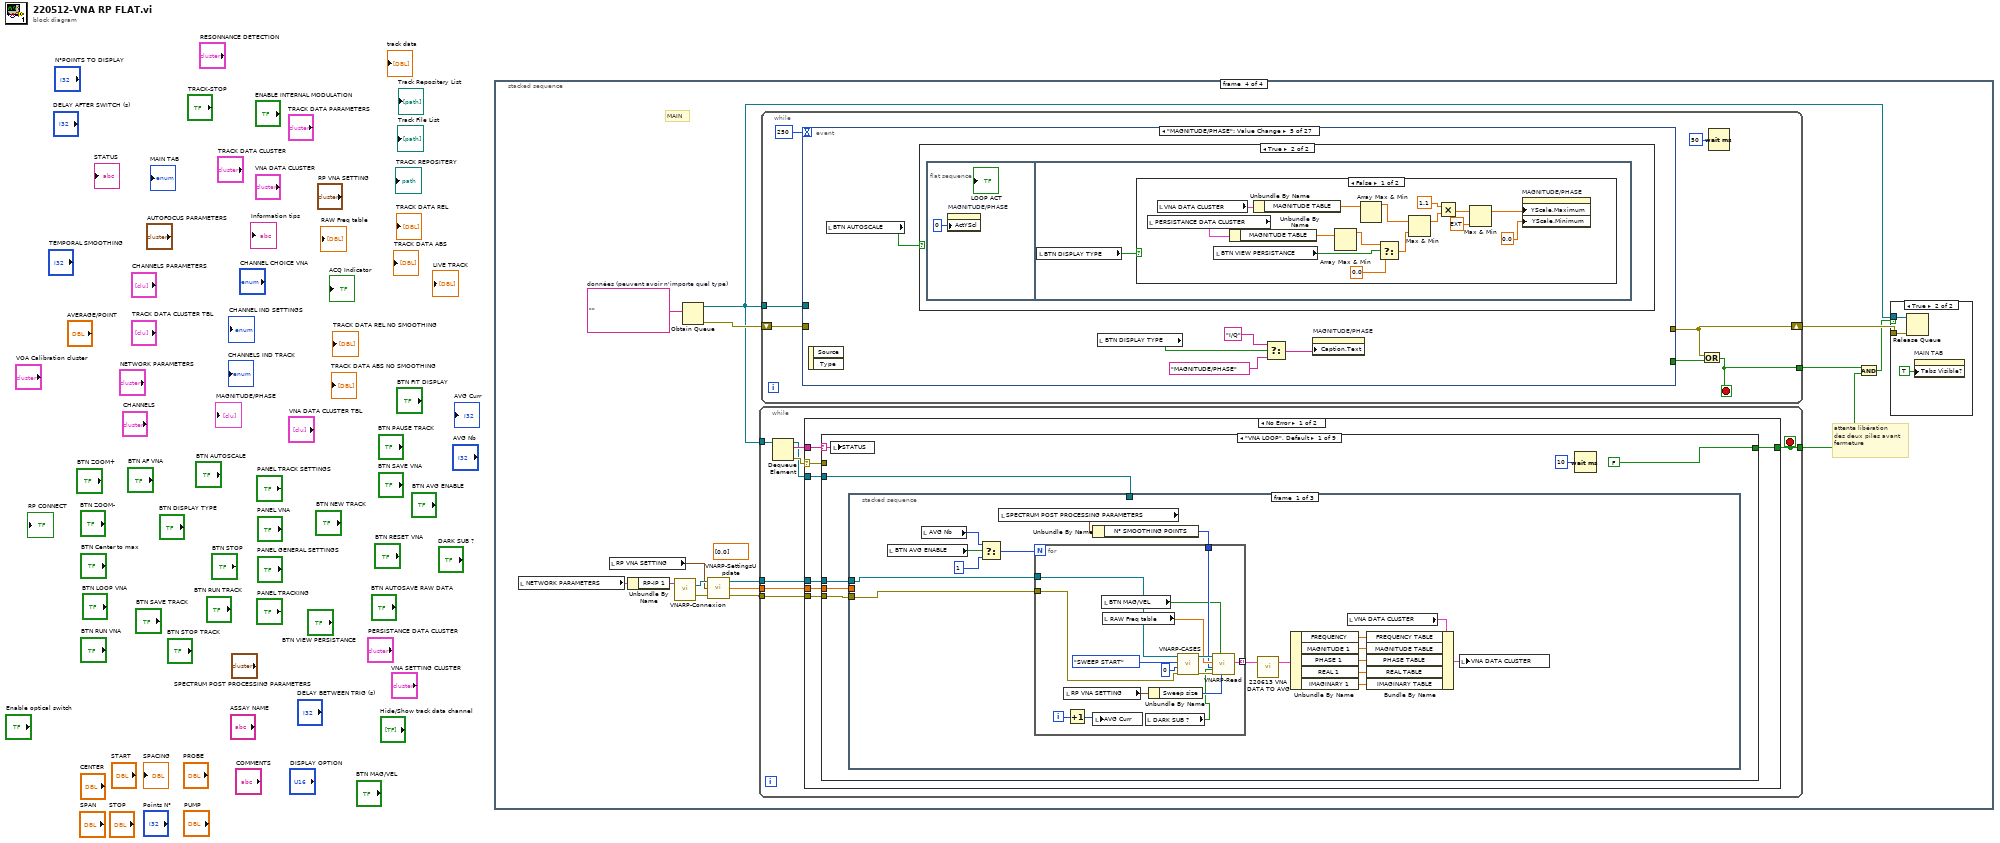
[diagram p0: block diagram]
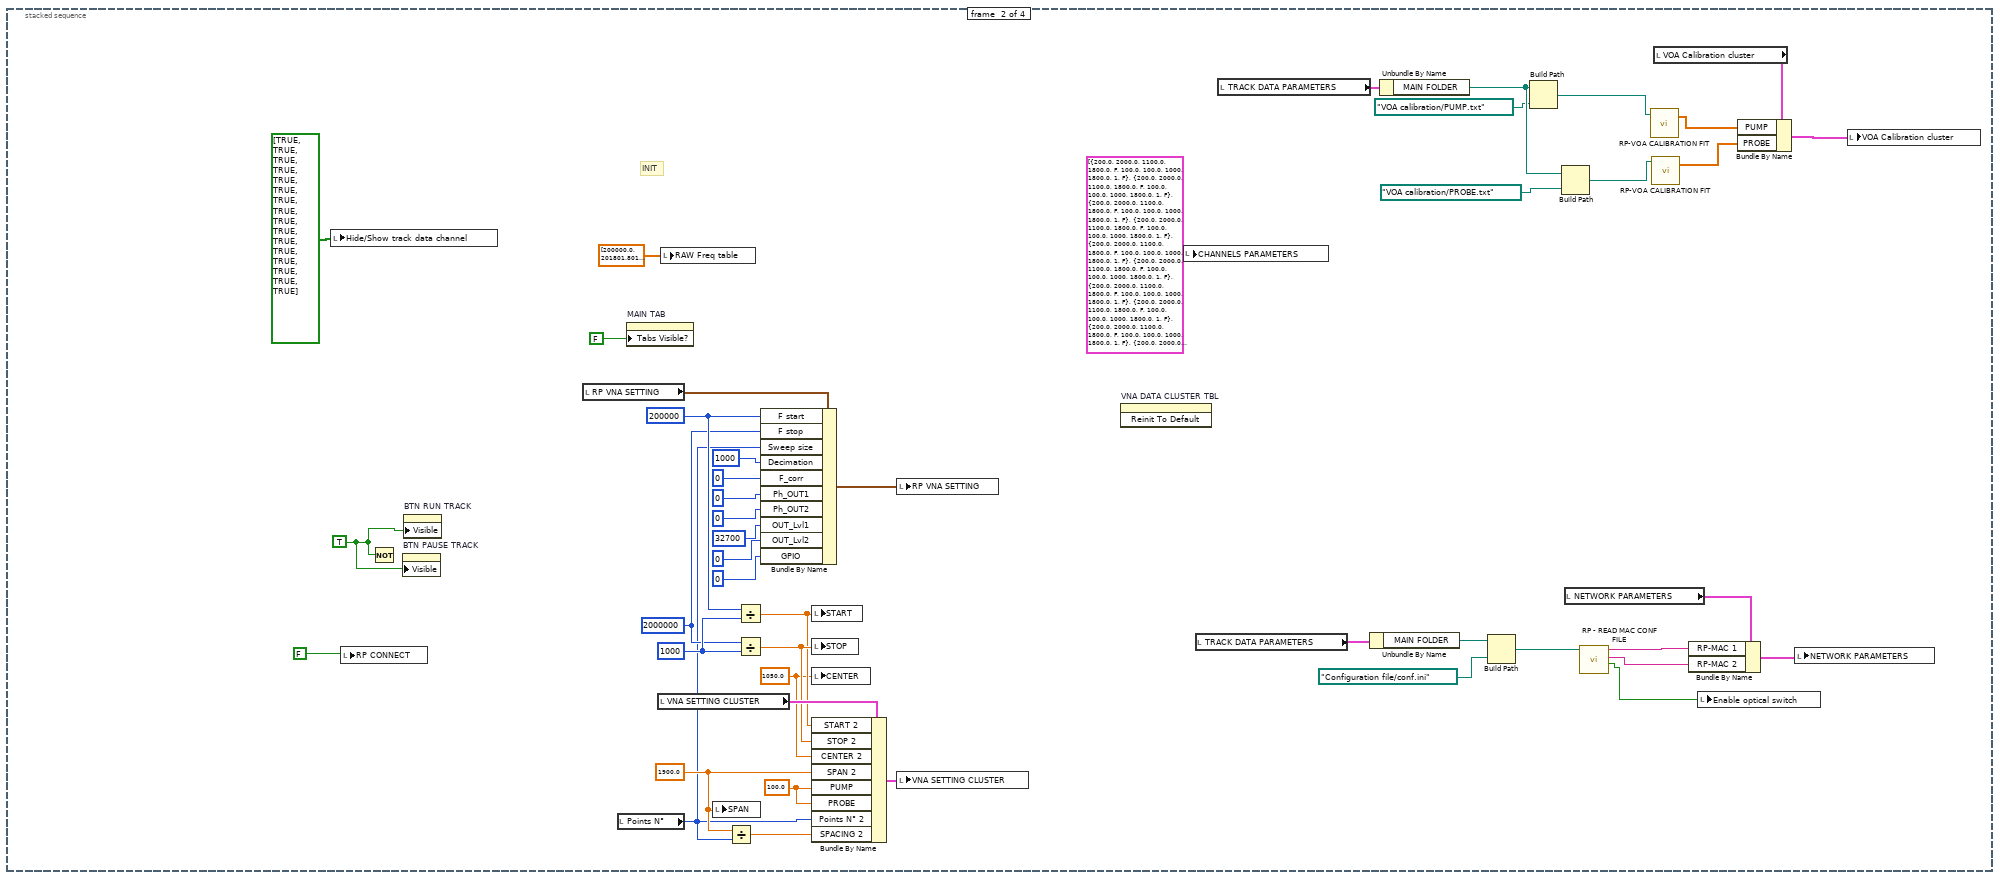
[diagram p3: hidden frame]
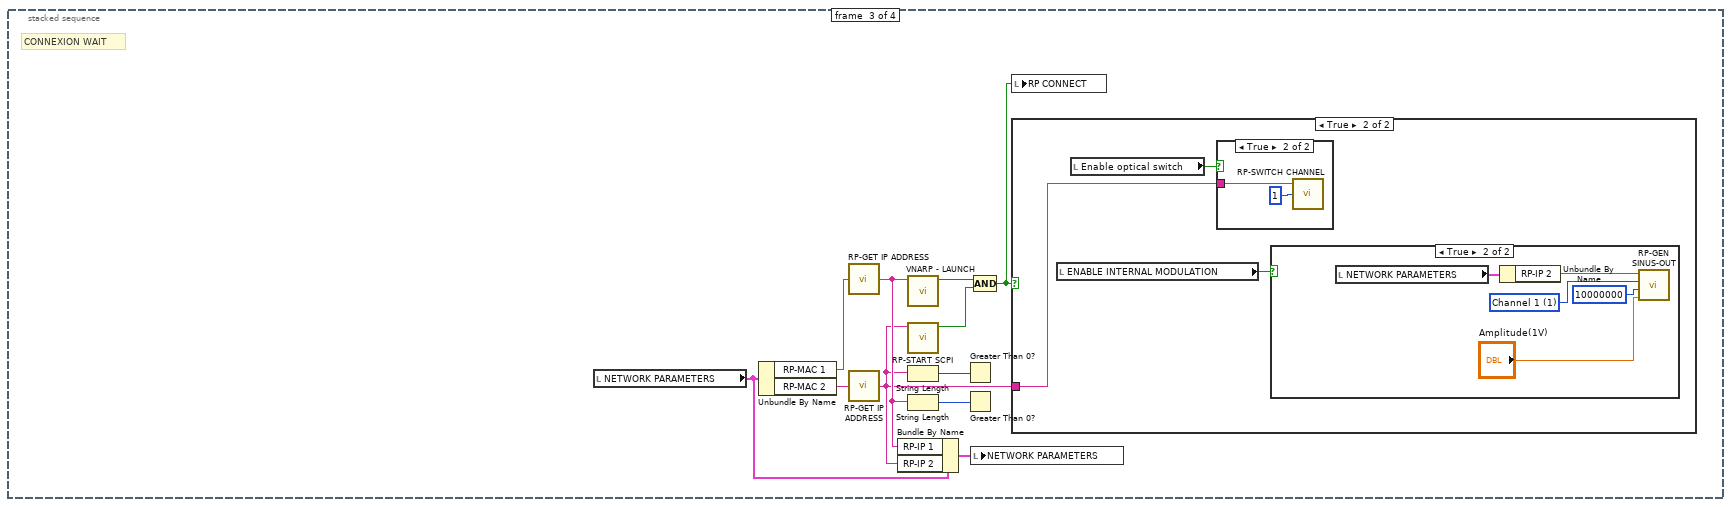
[diagram p4: hidden frame]
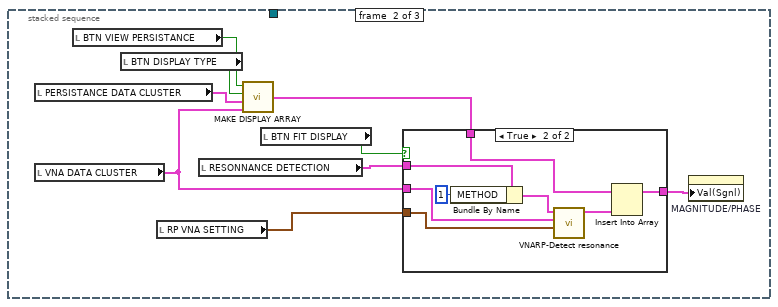
[diagram p9: hidden frame]
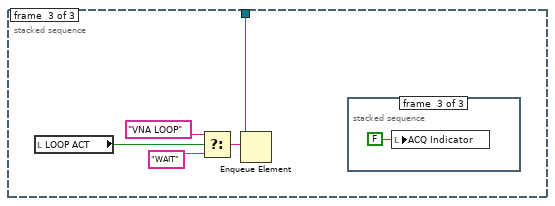
[diagram p11: hidden frame]
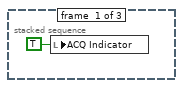
[diagram p12: hidden frame]
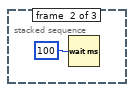
[diagram p13: hidden frame]
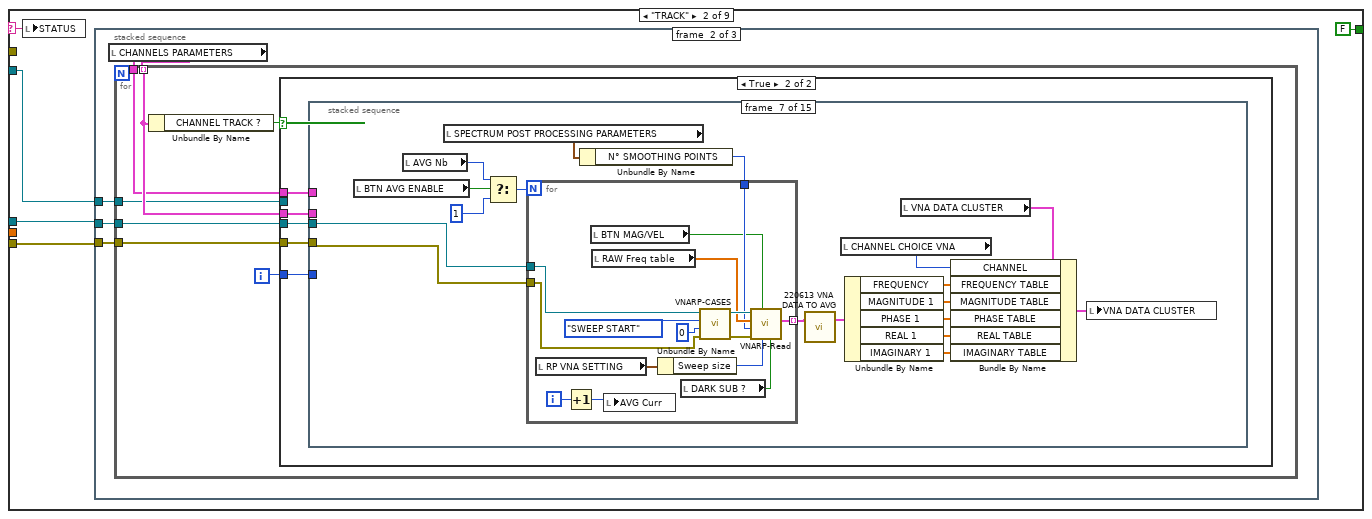
[diagram p14: hidden frame]
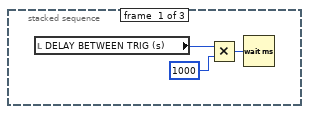
[diagram p15: hidden frame]
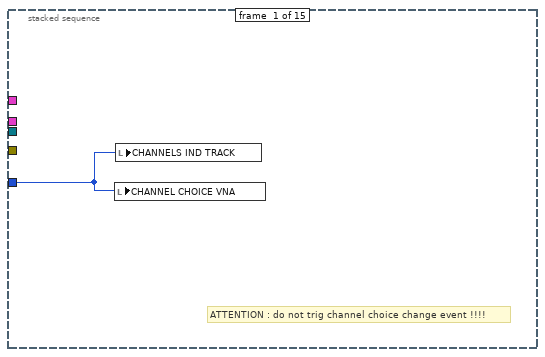
[diagram p17: hidden frame]
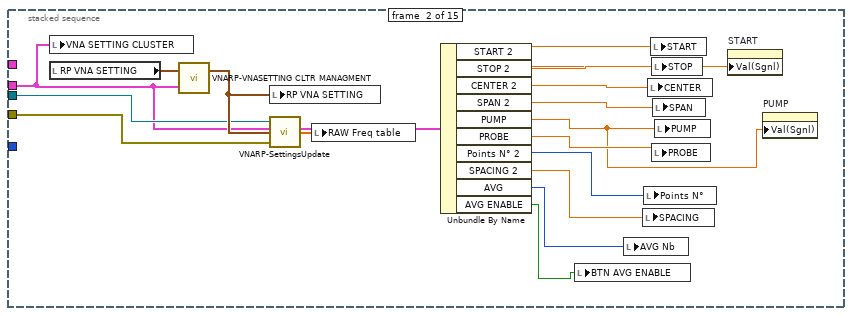
[diagram p18: hidden frame]
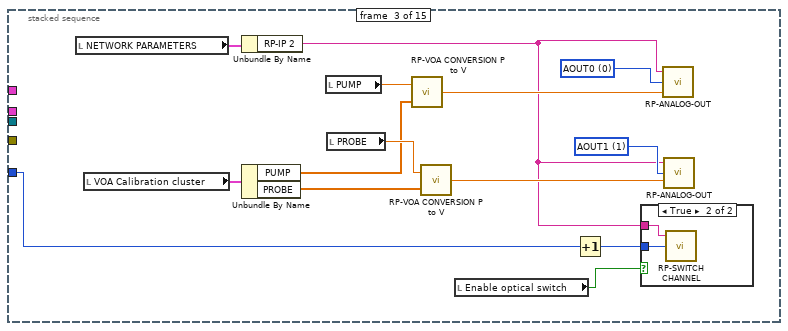
[diagram p19: hidden frame]
diagram:
  n1 = stacked-sequence {
    frame #0 {
    }
    frame #1 {
      w24 = TRUE ("x")
      w25 = 100.0 ("PUMP")
      w28 = 1900.0 ("Center")
      w29 = 1050.0 ("Center")
      w44 = u32 1000 ("Decimation")
      w42 = u32 2000000 ("Decimation")
      w43 = u32 200000 ("Decimation")
      # "INIT"
      n2 = local write "Hide/Show track data channel"(bool[] [TRUE, TRUE, TRUE, TRUE, TRUE, TRUE, TRUE, TRUE, TRUE, TRUE, TRUE, TRUE, TRUE, TRUE, TRUE, TRUE] ("Hide/Show track data channel")) -> ()
      n3 = local write "RP CONNECT"(FALSE) -> ()
      n4 = Not(x=w24) -> ()  [unwired: 1 out]
      n5 = property on="BTN PAUSE TRACK" class="Bool (strict)"("Visible"=w24) -> ()  [unwired: 2 in, 2 out]
      n6 = property on="BTN RUN TRACK" class="Bool (strict)"("Visible"=w24) -> ()  [unwired: 2 in, 2 out]
      n7 = local read "RP VNA SETTING"() -> (w46:T1)
      n8 = local read "Points N°"() -> (w27:i32)
      n9 = property on="MAIN TAB" class="TabCtl (strict)"("Tabs Visible?"=FALSE ("Onglets visibles ?")) -> ()  [unwired: 2 in, 2 out]
      n10 = local read "VNA SETTING CLUSTER"() -> (w33:T4)
      n11 = local write "RAW Freq table"(dbl[] [200000.0, 201801.8018018018, 203603.6036036036, 205405.4054054054, 207207.20720720722, 209009.009009009, 210810.8108108108, 212612.6126126126, 214414.4144144144, 216216.2162162162, 218018.01801801802, 219819.81981981982, 221621.62162162163, 223423.42342342343, 225225.22522522524, 227027.02702702704, 228828.82882882882, 230630.63063063062, 232432.43243243243, 234234.23423423423, 236036.03603603604, 237837.83783783784, 239639.63963963964, 241441.44144144145, 243243.24324324325, 245045.04504504503, 246846.84684684683, 248648.64864864864, 250450.45045045044, 252252.25225225225, 254054.05405405405, 255855.85585585586, 257657.65765765766, 259459.45945945947, 261261.26126126124, 263063.0630630631, 264864.86486486485, 266666.6666666666, 268468.46846846846, 270270.2702702703, 272072.0720720721, 273873.87387387385, 275675.6756756757, 277477.47747747746, 279279.2792792793, 281081.08108108107, 282882.8828828829, 284684.6846846847, 286486.4864864865, 288288.2882882883, 290090.09009009006, 291891.8918918919, 293693.69369369367, 295495.4954954955, 297297.2972972973, 299099.0990990991, 300900.9009009009, 302702.7027027027, 304504.5045045045, 306306.3063063063, 308108.1081081081, 309909.90990990994, 311711.7117117117, 313513.5135135135, 315315.3153153153, 317117.1171171171, 318918.91891891893, 320720.7207207207, 322522.5225225225, 324324.3243243243, 326126.12612612615, 327927.9279279279, 329729.7297297297, 331531.53153153154, 333333.3333333333, 335135.13513513515, 336936.9369369369, 338738.7387387387, 340540.54054054053, 342342.34234234237, 344144.14414414414, 345945.9459459459, 347747.74774774775, 349549.5495495496, 351351.35135135136, 353153.15315315314, 354954.9549549549, 356756.75675675675, 358558.5585585586, 360360.36036036036, 362162.16216216213, 363963.96396396396, 365765.7657657658, 367567.5675675676, 369369.36936936935, 371171.1711711711, 372972.97297297296, 374774.7747747748, 376576.57657657657, 378378.37837837834, 380180.1801801802, 381981.981981982, 383783.7837837838, 385585.58558558556, 387387.38738738734, 389189.1891891892, 390990.990990991, 392792.7927927928, 394594.59459459456, 396396.3963963964, 398198.1981981982, 400000.0, 401801.8018018018, 403603.6036036036, 405405.4054054054, 407207.2072072072, 409009.009009009, 410810.81081081077, 412612.6126126126, 414414.41441441444, 416216.2162162162, 418018.018018018, 419819.8198198198, 421621.62162162166, 423423.42342342343, 425225.2252252252, 427027.027027027, 428828.8288288288, 430630.63063063065, 432432.4324324324, 434234.2342342342, 436036.03603603604, 437837.83783783787, 439639.63963963964, 441441.4414414414, 443243.2432432432, 445045.04504504503, 446846.84684684686, 448648.64864864864, 450450.4504504504, 452252.25225225225, 454054.0540540541, 455855.85585585586, 457657.65765765763, 459459.4594594594, 461261.26126126124, 463063.0630630631, 464864.86486486485, 466666.6666666666, 468468.46846846846, 470270.27027027024, 472072.0720720721, 473873.87387387385, 475675.6756756757, 477477.47747747746, 479279.2792792793, 481081.08108108107, 482882.8828828829, 484684.6846846847, 486486.48648648645, 488288.2882882883, 490090.09009009006, 491891.8918918919, 493693.69369369367, 495495.4954954955, 497297.2972972973, 499099.0990990991, 500900.9009009009, 502702.70270270266, 504504.5045045045, 506306.3063063063, 508108.1081081081, 509909.9099099099, 511711.7117117117, 513513.5135135135, 515315.3153153153, 517117.1171171171, 518918.91891891893, 520720.7207207207, 522522.5225225225, 524324.3243243243, 526126.1261261262, 527927.9279279279, 529729.7297297297, 531531.5315315316, 533333.3333333333, 535135.1351351351, 536936.9369369369, 538738.7387387387, 540540.5405405406, 542342.3423423423, 544144.1441441441, 545945.9459459459, 547747.7477477477, 549549.5495495496, 551351.3513513514, 553153.1531531531, 554954.9549549549, 556756.7567567567, 558558.5585585586, 560360.3603603604, 562162.1621621621, 563963.963963964, 565765.7657657657, 567567.5675675676, 569369.3693693693, 571171.1711711711, 572972.972972973, 574774.7747747747, 576576.5765765766, 578378.3783783783, 580180.1801801801, 581981.981981982, 583783.7837837838, 585585.5855855856, 587387.3873873875, 589189.1891891891, 590990.990990991, 592792.7927927928, 594594.5945945946, 596396.3963963964, 598198.1981981981, 600000.0, 601801.8018018018, 603603.6036036036, 605405.4054054054, 607207.2072072072, 609009.009009009, 610810.8108108108, 612612.6126126125, 614414.4144144144, 616216.2162162162, 618018.018018018, 619819.8198198199, 621621.6216216215, 623423.4234234234, 625225.2252252252, 627027.027027027, 628828.8288288289, 630630.6306306305, 632432.4324324324, 634234.2342342342, 636036.036036036, 637837.8378378379, 639639.6396396396, 641441.4414414414, 643243.2432432433, 645045.045045045, 646846.8468468469, 648648.6486486486, 650450.4504504504, 652252.2522522523, 654054.054054054, 655855.8558558559, 657657.6576576576, 659459.4594594594, 661261.2612612613, 663063.063063063, 664864.8648648649, 666666.6666666666, 668468.4684684684, 670270.2702702703, 672072.0720720721, 673873.8738738738, 675675.6756756757, 677477.4774774774, 679279.2792792793, 681081.0810810811, 682882.8828828828, 684684.6846846847, 686486.4864864864, 688288.2882882883, 690090.0900900901, 691891.8918918918, 693693.6936936937, 695495.4954954955, 697297.2972972973, 699099.099099099, 700900.9009009008, 702702.7027027027, 704504.5045045045, 706306.3063063063, 708108.1081081082, 709909.9099099098, 711711.7117117117, 713513.5135135135, 715315.3153153153, 717117.1171171172, 718918.9189189188, 720720.7207207207, 722522.5225225225, 724324.3243243243, 726126.1261261262, 727927.9279279279, 729729.7297297297, 731531.5315315315, 733333.3333333333, 735135.1351351351, 736936.9369369369, 738738.7387387387, 740540.5405405405, 742342.3423423424, 744144.1441441441, 745945.9459459459, 747747.7477477477, 749549.5495495496, 751351.3513513514, 753153.1531531531, 754954.9549549549, 756756.7567567567, 758558.5585585586, 760360.3603603604, 762162.1621621621, 763963.9639639639, 765765.7657657658, 767567.5675675676, 769369.3693693693, 771171.1711711711, 772972.9729729729, 774774.7747747748, 776576.5765765766, 778378.3783783783, 780180.1801801801, 781981.981981982, 783783.7837837838, 785585.5855855856, 787387.3873873873, 789189.1891891891, 790990.990990991, 792792.7927927928, 794594.5945945946, 796396.3963963963, 798198.1981981982, 800000.0, 801801.8018018018, 803603.6036036036, 805405.4054054053, 807207.2072072072, 809009.009009009, 810810.8108108108, 812612.6126126125, 814414.4144144144, 816216.2162162162, 818018.018018018, 819819.8198198198, 821621.6216216215, 823423.4234234234, 825225.2252252252, 827027.027027027, 828828.8288288288, 830630.6306306307, 832432.4324324324, 834234.2342342342, 836036.036036036, 837837.8378378379, 839639.6396396396, 841441.4414414414, 843243.2432432432, 845045.045045045, 846846.8468468469, 848648.6486486486, 850450.4504504504, 852252.2522522522, 854054.0540540541, 855855.8558558559, 857657.6576576576, 859459.4594594594, 861261.2612612612, 863063.0630630631, 864864.8648648649, 866666.6666666666, 868468.4684684684, 870270.2702702703, 872072.0720720721, 873873.8738738738, 875675.6756756756, 877477.4774774774, 879279.2792792793, 881081.0810810811, 882882.8828828828, 884684.6846846846, 886486.4864864865, 888288.2882882883, 890090.0900900901, 891891.8918918918, 893693.6936936936, 895495.4954954955, 897297.2972972973, 899099.099099099, 900900.9009009008, 902702.7027027027, 904504.5045045045, 906306.3063063063, 908108.108108108, 909909.9099099098, 911711.7117117117, 913513.5135135135, 915315.3153153153, 917117.117117117, 918918.9189189189, 920720.7207207207, 922522.5225225225, 924324.3243243243, 926126.1261261262, 927927.9279279279, 929729.7297297297, 931531.5315315315, 933333.3333333333, 935135.1351351351, 936936.9369369369, 938738.7387387387, 940540.5405405405, 942342.3423423424, 944144.1441441441, 945945.9459459459, 947747.7477477477, 949549.5495495495, 951351.3513513514, 953153.1531531531, 954954.9549549549, 956756.7567567567, 958558.5585585586, 960360.3603603604, 962162.1621621621, 963963.9639639639, 965765.7657657657, 967567.5675675676, 969369.3693693693, 971171.1711711711, 972972.9729729729, 974774.7747747748, 976576.5765765766, 978378.3783783783, 980180.1801801801, 981981.9819819819, 983783.7837837838, 985585.5855855856, 987387.3873873873, 989189.1891891891, 990990.990990991, 992792.7927927928, 994594.5945945946, 996396.3963963963, 998198.1981981982, 1000000.0, 1001801.8018018018, 1003603.6036036036, 1005405.4054054053, 1007207.2072072072, 1009009.009009009, 1010810.8108108108, 1012612.6126126125, 1014414.4144144144, 1016216.2162162162, 1018018.018018018, 1019819.8198198198, 1021621.6216216215, 1023423.4234234234, 1025225.2252252252, 1027027.027027027, 1028828.8288288288, 1030630.6306306307, 1032432.4324324324, 1034234.2342342342, 1036036.036036036, 1037837.8378378378, 1039639.6396396396, 1041441.4414414414, 1043243.2432432432, 1045045.045045045, 1046846.8468468469, 1048648.6486486485, 1050450.4504504504, 1052252.2522522523, 1054054.054054054, 1055855.8558558559, 1057657.6576576577, 1059459.4594594594, 1061261.261261261, 1063063.0630630632, 1064864.8648648649, 1066666.6666666665, 1068468.4684684684, 1070270.2702702703, 1072072.072072072, 1073873.8738738738, 1075675.6756756757, 1077477.4774774774, 1079279.2792792793, 1081081.0810810812, 1082882.8828828828, 1084684.6846846845, 1086486.4864864866, 1088288.2882882883, 1090090.09009009, 1091891.8918918918, 1093693.6936936937, 1095495.4954954954, 1097297.2972972973, 1099099.0990990992, 1100900.9009009008, 1102702.7027027027, 1104504.5045045046, 1106306.3063063063, 1108108.108108108, 1109909.9099099098, 1111711.7117117117, 1113513.5135135134, 1115315.3153153153, 1117117.1171171172, 1118918.9189189188, 1120720.7207207207, 1122522.5225225226, 1124324.3243243243, 1126126.126126126, 1127927.927927928, 1129729.7297297297, 1131531.5315315314, 1133333.3333333333, 1135135.1351351351, 1136936.9369369368, 1138738.7387387387, 1140540.5405405406, 1142342.3423423423, 1144144.1441441441, 1145945.945945946, 1147747.7477477477, 1149549.5495495494, 1151351.3513513515, 1153153.1531531531, 1154954.9549549548, 1156756.7567567567, 1158558.5585585586, 1160360.3603603602, 1162162.1621621621, 1163963.963963964, 1165765.7657657657, 1167567.5675675676, 1169369.3693693695, 1171171.1711711711, 1172972.9729729728, 1174774.774774775, 1176576.5765765766, 1178378.3783783782, 1180180.1801801801, 1181981.981981982, 1183783.7837837837, 1185585.5855855856, 1187387.3873873875, 1189189.189189189, 1190990.990990991, 1192792.792792793, 1194594.5945945946, 1196396.3963963962, 1198198.198198198, 1200000.0, 1201801.8018018017, 1203603.6036036036, 1205405.4054054054, 1207207.207207207, 1209009.009009009, 1210810.810810811, 1212612.6126126125, 1214414.4144144142, 1216216.2162162163, 1218018.018018018, 1219819.8198198196, 1221621.6216216215, 1223423.4234234234, 1225225.225225225, 1227027.027027027, 1228828.8288288289, 1230630.6306306305, 1232432.4324324324, 1234234.2342342343, 1236036.036036036, 1237837.8378378376, 1239639.6396396398, 1241441.4414414414, 1243243.243243243, 1245045.045045045, 1246846.8468468469, 1248648.6486486485, 1250450.4504504504, 1252252.2522522523, 1254054.054054054, 1255855.8558558559, 1257657.6576576575, 1259459.4594594594, 1261261.2612612613, 1263063.063063063, 1264864.8648648649, 1266666.6666666665, 1268468.4684684684, 1270270.2702702703, 1272072.072072072, 1273873.8738738738, 1275675.6756756757, 1277477.4774774774, 1279279.2792792793, 1281081.081081081, 1282882.8828828828, 1284684.6846846847, 1286486.4864864864, 1288288.2882882883, 1290090.09009009, 1291891.8918918918, 1293693.6936936937, 1295495.4954954954, 1297297.2972972973, 1299099.0990990992, 1300900.9009009008, 1302702.7027027027, 1304504.5045045044, 1306306.3063063063, 1308108.1081081082, 1309909.9099099098, 1311711.7117117117, 1313513.5135135134, 1315315.3153153153, 1317117.1171171172, 1318918.9189189188, 1320720.7207207207, 1322522.5225225224, 1324324.3243243243, 1326126.1261261262, 1327927.9279279278, 1329729.7297297297, 1331531.5315315316, 1333333.3333333333, 1335135.1351351351, 1336936.9369369368, 1338738.7387387387, 1340540.5405405406, 1342342.3423423423, 1344144.1441441441, 1345945.9459459458, 1347747.7477477477, 1349549.5495495496, 1351351.3513513512, 1353153.1531531531, 1354954.9549549548, 1356756.7567567567, 1358558.5585585586, 1360360.3603603602, 1362162.1621621621, 1363963.963963964, 1365765.7657657657, 1367567.5675675676, 1369369.3693693692, 1371171.1711711711, 1372972.972972973, 1374774.7747747747, 1376576.5765765766, 1378378.3783783782, 1380180.1801801801, 1381981.981981982, 1383783.7837837837, 1385585.5855855856, 1387387.3873873875, 1389189.189189189, 1390990.990990991, 1392792.7927927927, 1394594.5945945946, 1396396.3963963964, 1398198.198198198, 1400000.0, 1401801.8018018017, 1403603.6036036036, 1405405.4054054054, 1407207.207207207, 1409009.009009009, 1410810.8108108107, 1412612.6126126125, 1414414.4144144144, 1416216.216216216, 1418018.018018018, 1419819.8198198199, 1421621.6216216215, 1423423.4234234234, 1425225.225225225, 1427027.027027027, 1428828.8288288289, 1430630.6306306305, 1432432.4324324324, 1434234.234234234, 1436036.036036036, 1437837.8378378379, 1439639.6396396395, 1441441.4414414414, 1443243.243243243, 1445045.045045045, 1446846.8468468469, 1448648.6486486485, 1450450.4504504504, 1452252.2522522523, 1454054.054054054, 1455855.8558558559, 1457657.6576576575, 1459459.4594594594, 1461261.2612612613, 1463063.063063063, 1464864.8648648649, 1466666.6666666665, 1468468.4684684684, 1470270.2702702703, 1472072.072072072, 1473873.8738738738, 1475675.6756756757, 1477477.4774774774, 1479279.2792792793, 1481081.081081081, 1482882.8828828828, 1484684.6846846847, 1486486.4864864864, 1488288.2882882883, 1490090.09009009, 1491891.8918918918, 1493693.6936936937, 1495495.4954954954, 1497297.2972972973, 1499099.099099099, 1500900.9009009008, 1502702.7027027027, 1504504.5045045044, 1506306.3063063063, 1508108.1081081082, 1509909.9099099098, 1511711.7117117117, 1513513.5135135134, 1515315.3153153153, 1517117.1171171172, 1518918.9189189188, 1520720.7207207207, 1522522.5225225224, 1524324.3243243243, 1526126.1261261262, 1527927.9279279278, 1529729.7297297297, 1531531.5315315314, 1533333.3333333333, 1535135.1351351351, 1536936.9369369368, 1538738.7387387387, 1540540.5405405406, 1542342.3423423423, 1544144.1441441441, 1545945.9459459458, 1547747.7477477477, 1549549.5495495496, 1551351.3513513512, 1553153.1531531531, 1554954.9549549548, 1556756.7567567567, 1558558.5585585586, 1560360.3603603602, 1562162.1621621621, 1563963.963963964, 1565765.7657657657, 1567567.5675675676, 1569369.3693693692, 1571171.1711711711, 1572972.972972973, 1574774.7747747747, 1576576.5765765766, 1578378.3783783782, 1580180.1801801801, 1581981.981981982, 1583783.7837837837, 1585585.5855855856, 1587387.3873873872, 1589189.189189189, 1590990.990990991, 1592792.7927927927, 1594594.5945945946, 1596396.3963963964, 1598198.198198198, 1600000.0, 1601801.8018018017, 1603603.6036036036, 1605405.4054054054, 1607207.207207207, 1609009.009009009, 1610810.8108108107, 1612612.6126126125, 1614414.4144144144, 1616216.216216216, 1618018.018018018, 1619819.8198198196, 1621621.6216216215, 1623423.4234234234, 1625225.225225225, 1627027.027027027, 1628828.8288288289, 1630630.6306306305, 1632432.4324324324, 1634234.234234234, 1636036.036036036, 1637837.8378378379, 1639639.6396396395, 1641441.4414414414, 1643243.243243243, 1645045.045045045, 1646846.8468468469, 1648648.6486486485, 1650450.4504504504, 1652252.2522522523, 1654054.054054054, 1655855.8558558559, 1657657.6576576575, 1659459.4594594594, 1661261.2612612613, 1663063.063063063, 1664864.8648648649, 1666666.6666666665, 1668468.4684684684, 1670270.2702702703, 1672072.072072072, 1673873.8738738738, 1675675.6756756755, 1677477.4774774774, 1679279.2792792793, 1681081.081081081, 1682882.8828828828, 1684684.6846846847, 1686486.4864864864, 1688288.2882882883, 1690090.09009009, 1691891.8918918918, 1693693.6936936937, 1695495.4954954954, 1697297.2972972973, 1699099.099099099, 1700900.9009009008, 1702702.7027027027, 1704504.5045045044, 1706306.3063063063, 1708108.108108108, 1709909.9099099098, 1711711.7117117117, 1713513.5135135134, 1715315.3153153153, 1717117.1171171172, 1718918.9189189188, 1720720.7207207207, 1722522.5225225224, 1724324.3243243243, 1726126.1261261262, 1727927.9279279278, 1729729.7297297297, 1731531.5315315314, 1733333.3333333333, 1735135.1351351351, 1736936.9369369368, 1738738.7387387387, 1740540.5405405406, 1742342.3423423423, 1744144.1441441441, 1745945.9459459458, 1747747.7477477477, 1749549.5495495496, 1751351.3513513512, 1753153.1531531531, 1754954.9549549548, 1756756.7567567567, 1758558.5585585586, 1760360.3603603602, 1762162.1621621621, 1763963.9639639638, 1765765.7657657657, 1767567.5675675676, 1769369.3693693692, 1771171.1711711711, 1772972.972972973, 1774774.7747747747, 1776576.5765765766, 1778378.3783783782, 1780180.1801801801, 1781981.981981982, 1783783.7837837837, 1785585.5855855856, 1787387.3873873872, 1789189.189189189, 1790990.990990991, 1792792.7927927927, 1794594.5945945946, 1796396.3963963964, 1798198.198198198, 1800000.0, 1801801.8018018017, 1803603.6036036036, 1805405.4054054054, 1807207.207207207, 1809009.009009009, 1810810.8108108107, 1812612.6126126125, 1814414.4144144144, 1816216.216216216, 1818018.018018018, 1819819.8198198196, 1821621.6216216215, 1823423.4234234234, 1825225.225225225, 1827027.027027027, 1828828.8288288289, 1830630.6306306305, 1832432.4324324324, 1834234.234234234, 1836036.036036036, 1837837.8378378379, 1839639.6396396395, 1841441.4414414414, 1843243.243243243, 1845045.045045045, 1846846.8468468469, 1848648.6486486485, 1850450.4504504504, 1852252.252252252, 1854054.054054054, 1855855.8558558559, 1857657.6576576575, 1859459.4594594594, 1861261.2612612613, 1863063.063063063, 1864864.8648648649, 1866666.6666666665, 1868468.4684684684, 1870270.2702702703, 1872072.072072072, 1873873.8738738738, 1875675.6756756755, 1877477.4774774774, 1879279.2792792793, 1881081.081081081, 1882882.8828828828, 1884684.6846846847, 1886486.4864864864, 1888288.2882882883, 1890090.09009009, 1891891.8918918918, 1893693.6936936937, 1895495.4954954954, 1897297.2972972973, 1899099.099099099, 1900900.9009009008, 1902702.7027027027, 1904504.5045045044, 1906306.3063063063, 1908108.108108108, 1909909.9099099098, 1911711.7117117117, 1913513.5135135134, 1915315.3153153153, 1917117.1171171172, 1918918.9189189188, 1920720.7207207207, 1922522.5225225224, 1924324.3243243243, 1926126.1261261262, 1927927.9279279278, 1929729.7297297297, 1931531.5315315314, 1933333.3333333333, 1935135.1351351351, 1936936.9369369368, 1938738.7387387387, 1940540.5405405404, 1942342.3423423423, 1944144.1441441441, 1945945.9459459458, 1947747.7477477477, 1949549.5495495496, 1951351.3513513512, 1953153.1531531531, 1954954.9549549548, 1956756.7567567567, 1958558.5585585586, 1960360.3603603602, 1962162.1621621621, 1963963.9639639638, 1965765.7657657657, 1967567.5675675676, 1969369.3693693692, 1971171.1711711711, 1972972.972972973, 1974774.7747747747, 1976576.5765765766, 1978378.3783783782, 1980180.1801801801, 1981981.981981982, 1983783.7837837837, 1985585.5855855856, 1987387.3873873872, 1989189.189189189, 1990990.990990991, 1992792.7927927927, 1994594.5945945946, 1996396.3963963962, 1998198.198198198, 2000000.0] ("RAW Freq table")) -> ()
      n12 = local write "SPAN"(w28) -> ()
      n13 = Divide(x=w28, y=w27) -> (x/y=w26:dbl)
      n14 = Divide(x=w43, y=w44) -> (x/y=w30:dbl)
      n15 = Divide(x=w42, y=w44) -> (x/y=w31:dbl)
      n16 = Bundle By Name(cluster=w46, "F start"=w43, "F stop"=w42, "Sweep size"=w27, "Decimation"=u32 1000, "F_corr"=u32 0, "Ph_OUT1"=u32 0, "Ph_OUT2"=u32 0 ("F_corr"), "OUT_Lvl1"=u32 32700 ("F_corr"), "OUT_Lvl2"=u32 0 ("F_corr"), "GPIO"=u32 0 ("F_corr")) -> (w45:T1)
      n17 = local write "START"(w30) -> ()
      n18 = local write "STOP"(w31) -> ()
      n19 = local write "CENTER"(w29) -> ()
      n20 = Bundle By Name(cluster=w33, "START 2"=w30, "STOP 2"=w31, "CENTER 2"=w29, "SPAN 2"=w28, "PUMP"=w25, "PROBE"=w25, "Points N° 2"=w27, "SPACING 2"=w26) -> (w32:T4)
      n21 = local write "RP VNA SETTING"(w45) -> ()
      n22 = local write "VNA SETTING CLUSTER"(w32) -> ()
      n23 = invoke on="VNA DATA CLUSTER TBL" class="Arr (strict)" method="Reinit To Default"() -> ()  [unwired: 3 in, 3 out]
      n24 = local write "CHANNELS PARAMETERS"(T4[] [{"START 2"=200.0, "STOP 2"=2000.0, "CENTER 2"=1100.0, "SPAN 2"=1800.0, "CHANNEL TRACK ?"=FALSE, "PUMP"=100.0, "PROBE"=100.0, "Points N° 2"=1000, "SPACING 2"=1800.0, "AVG"=1, "AVG ENABLE"=FALSE}, {"START 2"=200.0, "STOP 2"=2000.0, "CENTER 2"=1100.0, "SPAN 2"=1800.0, "CHANNEL TRACK ?"=FALSE, "PUMP"=100.0, "PROBE"=100.0, "Points N° 2"=1000, "SPACING 2"=1800.0, "AVG"=1, "AVG ENABLE"=FALSE}, {"START 2"=200.0, "STOP 2"=2000.0, "CENTER 2"=1100.0, "SPAN 2"=1800.0, "CHANNEL TRACK ?"=FALSE, "PUMP"=100.0, "PROBE"=100.0, "Points N° 2"=1000, "SPACING 2"=1800.0, "AVG"=1, "AVG ENABLE"=FALSE}, {"START 2"=200.0, "STOP 2"=2000.0, "CENTER 2"=1100.0, "SPAN 2"=1800.0, "CHANNEL TRACK ?"=FALSE, "PUMP"=100.0, "PROBE"=100.0, "Points N° 2"=1000, "SPACING 2"=1800.0, "AVG"=1, "AVG ENABLE"=FALSE}, {"START 2"=200.0, "STOP 2"=2000.0, "CENTER 2"=1100.0, "SPAN 2"=1800.0, "CHANNEL TRACK ?"=FALSE, "PUMP"=100.0, "PROBE"=100.0, "Points N° 2"=1000, "SPACING 2"=1800.0, "AVG"=1, "AVG ENABLE"=FALSE}, {"START 2"=200.0, "STOP 2"=2000.0, "CENTER 2"=1100.0, "SPAN 2"=1800.0, "CHANNEL TRACK ?"=FALSE, "PUMP"=100.0, "PROBE"=100.0, "Points N° 2"=1000, "SPACING 2"=1800.0, "AVG"=1, "AVG ENABLE"=FALSE}, {"START 2"=200.0, "STOP 2"=2000.0, "CENTER 2"=1100.0, "SPAN 2"=1800.0, "CHANNEL TRACK ?"=FALSE, "PUMP"=100.0, "PROBE"=100.0, "Points N° 2"=1000, "SPACING 2"=1800.0, "AVG"=1, "AVG ENABLE"=FALSE}, {"START 2"=200.0, "STOP 2"=2000.0, "CENTER 2"=1100.0, "SPAN 2"=1800.0, "CHANNEL TRACK ?"=FALSE, "PUMP"=100.0, "PROBE"=100.0, "Points N° 2"=1000, "SPACING 2"=1800.0, "AVG"=1, "AVG ENABLE"=FALSE}, {"START 2"=200.0, "STOP 2"=2000.0, "CENTER 2"=1100.0, "SPAN 2"=1800.0, "CHANNEL TRACK ?"=FALSE, "PUMP"=100.0, "PROBE"=100.0, "Points N° 2"=1000, "SPACING 2"=1800.0, "AVG"=1, "AVG ENABLE"=FALSE}, {"START 2"=200.0, "STOP 2"=2000.0, "CENTER 2"=1100.0, "SPAN 2"=1800.0, "CHANNEL TRACK ?"=FALSE, "PUMP"=100.0, "PROBE"=100.0, "Points N° 2"=1000, "SPACING 2"=1800.0, "AVG"=1, "AVG ENABLE"=FALSE}, {"START 2"=200.0, "STOP 2"=2000.0, "CENTER 2"=1100.0, "SPAN 2"=1800.0, "CHANNEL TRACK ?"=FALSE, "PUMP"=100.0, "PROBE"=100.0, "Points N° 2"=1000, "SPACING 2"=1800.0, "AVG"=1, "AVG ENABLE"=FALSE}, {"START 2"=200.0, "STOP 2"=2000.0, "CENTER 2"=1100.0, "SPAN 2"=1800.0, "CHANNEL TRACK ?"=FALSE, "PUMP"=100.0, "PROBE"=100.0, "Points N° 2"=1000, "SPACING 2"=1800.0, "AVG"=1, "AVG ENABLE"=FALSE}, {"START 2"=200.0, "STOP 2"=2000.0, "CENTER 2"=1100.0, "SPAN 2"=1800.0, "CHANNEL TRACK ?"=FALSE, "PUMP"=100.0, "PROBE"=100.0, "Points N° 2"=1000, "SPACING 2"=1800.0, "AVG"=1, "AVG ENABLE"=FALSE}, {"START 2"=200.0, "STOP 2"=2000.0, "CENTER 2"=1100.0, "SPAN 2"=1800.0, "CHANNEL TRACK ?"=FALSE, "PUMP"=100.0, "PROBE"=100.0, "Points N° 2"=1000, "SPACING 2"=1800.0, "AVG"=1, "AVG ENABLE"=FALSE}, {"START 2"=200.0, "STOP 2"=2000.0, "CENTER 2"=1100.0, "SPAN 2"=1800.0, "CHANNEL TRACK ?"=FALSE, "PUMP"=100.0, "PROBE"=100.0, "Points N° 2"=1000, "SPACING 2"=1800.0, "AVG"=1, "AVG ENABLE"=FALSE}, {"START 2"=200.0, "STOP 2"=2000.0, "CENTER 2"=1100.0, "SPAN 2"=1800.0, "CHANNEL TRACK ?"=FALSE, "PUMP"=100.0, "PROBE"=100.0, "Points N° 2"=1000, "SPACING 2"=1800.0, "AVG"=1, "AVG ENABLE"=FALSE}] ("CHANNELS PARAMETERS")) -> ()
      n25 = local read "TRACK DATA PARAMETERS"() -> (w20:cluster{"MAIN FOLDER":path})
      n26 = local read "TRACK DATA PARAMETERS"() -> (w5:cluster{"MAIN FOLDER":path})
      n27 = Unbundle By Name(w20) -> ("MAIN FOLDER"=w19:path)
      n28 = Unbundle By Name(w5) -> ("MAIN FOLDER"=w6:path)
      n29 = Build Path(base path=w19, name or relative path=path "Configuration file/conf.ini") -> (appended path=w17:path)
      n30 = Build Path(base path=w6, name or relative path=path "VOA calibration/PUMP.txt") -> (appended path=w9:path)
      n31 = Build Path(base path=w6, name or relative path=path "VOA calibration/PROBE.txt") -> (appended path=w10:path)
      n32 = local read "NETWORK PARAMETERS"() -> (w16:T8)
      n33 = call "RP - READ MAC CONF FILE.vi"("Path"=w17) -> ("Activate switch"=w2:bool, "RP2 MAC"=w14:string, "RP1 MAC"=w15:string)  [unwired: 7 in, 1 out]
      n34 = call "RP-VOA CALIBRATION FIT.vi"("file path"=w9) -> ("Calibration array"=w11:dbl[])  [unwired: 2 in, 1 out]
      n35 = call "RP-VOA CALIBRATION FIT.vi"("file path"=w10) -> ("Calibration array"=w12:dbl[])  [unwired: 2 in, 1 out]
      n36 = local read "VOA Calibration cluster"() -> (w7:cluster{"PUMP":dbl[], "PROBE":dbl[]})
      n37 = Bundle By Name(cluster=w16, "RP-MAC 1"=w15, "RP-MAC 2"=w14) -> (w13:T8)
      n38 = local write "Enable optical switch"(w2) -> ()
      n39 = Bundle By Name(cluster=w7, "PUMP"=w11, "PROBE"=w12) -> (w8:cluster{"PUMP":dbl[], "PROBE":dbl[]})
      n40 = local write "NETWORK PARAMETERS"(w13) -> ()
      n41 = local write "VOA Calibration cluster"(w8) -> ()
    }
    frame #2 {
      # "CONNEXION WAIT"
      n42 = local read "NETWORK PARAMETERS"() -> (w51:T8)
      n43 = Unbundle By Name(w51) -> ("RP-MAC 1"=w50:string, "RP-MAC 2"=w49:string)
      n44 = call "RP-GET IP ADDRESS.vi"("MAC address"=w50) -> ("IP address"=w53:string)
      n45 = call "RP-GET IP ADDRESS.vi"("MAC address"=w49) -> ("IP address"=w47:string)
      n46 = Bundle By Name(cluster=w51, "RP-IP 1"=w53, "RP-IP 2"=w47) -> (w57:T8)
      n47 = call "VNARP - LAUNCH.vi"("RP IP"=w53) -> ("VNA launched ?"=w54:bool)  [unwired: 10 in]
      n48 = call "RP-START SCPI.vi"("RP IP"=w47) -> ("SCPI launched ?"=w52:bool)  [unwired: 10 in]
      n49 = String Length(string=w47) -> (length=w56:i32)
      n50 = String Length(string=w53) -> (length=w55:i32)
      n51 = Greater Than 0?(x=w56) -> ()  [unwired: 1 out]
      n52 = Greater Than 0?(x=w55) -> ()  [unwired: 1 out]
      n53 = local write "NETWORK PARAMETERS"(w57) -> ()
      n54 = Compound Arithmetic op=AND(w54, w52) -> (w48:bool)
      n55 = local write "RP CONNECT"(w48) -> ()
      n56 = case shown="True" w48 {
        tunnel: w47 -> [_ w59]
        frame False {
        }
        frame True {
          n57 = local read "ENABLE INTERNAL MODULATION"() -> (w60:bool)
          n58 = local read "Enable optical switch"() -> (w58:bool)
          n59 = case shown="True" w58 {
            tunnel: w59 -> [_ w62]
            frame False {
            }
            frame True {
              n60 = call "RP-SWITCH CHANNEL.vi"("Channel"=1, "IP address"=w62) -> ()  [unwired: 1 in, 2 out]
            }
          }
          n61 = case shown="True" w60 {
            frame False {
            }
            frame True {
              w65 = u16 1 items=["Channel 1"=1, "Channel 2"=2] ("Channel (1|2)")
              n62 = local read "NETWORK PARAMETERS"() -> (w64:T8)
              n63 = Unbundle By Name(w64) -> ("RP-IP 2"=w63:string)
              n64 = call "RP-GEN SINUS-OUT.vi"("Amplitude(1V)"="Amplitude(1V)", "Frequency (Hz)"=10000000, "Channel (1|2)"=w65, "IP address"=w63) -> ()  [unwired: 1 out]
            }
          }
        }
      }
    }
    frame #3 {
      (unwired) dbl[] [0.0]
      w80 = ""  # données (peuvent avoir n'importe quel type)
      # "attente libération des deux piles avant fermeture"
      # "MAIN"
      n65 = local read "NETWORK PARAMETERS"() -> (w69:T8)
      n66 = local read "RP VNA SETTING"() -> (w76:T1)
      n67 = Unbundle By Name(w69) -> ("RP-IP 1"=w68:string)
      n68 = call "VNARP-Connexion.vi"("IP RP"=w68) -> ("sortie d'erreur"=w78:errorcluster, "ID de connexion"=w77:refnum<k5>)  [unwired: 1 in]
      n69 = Obtain Queue(element data type=w80) -> (queue out=w79:refnum<queue>, error out=w82:errorcluster)  [unwired: 4 in, 1 out]
      n70 = call "VNARP-SettingsUpdate.vi"("Error IN"=w78, "RP VNA SETTINGS IN"=w76, "ID de connexion IN"=w77) -> ("Error OUT"=w73:errorcluster, "Freq table"=w74:dbl[], "ID de connexion OUT"=w75:refnum<k5>)
      n71 = while {
        tunnel: w79 -> [w91]
        tunnel: w75 -> [w89]
        tunnel: w74 -> [w88]
        tunnel: w73 -> [w87]
        tunnel: [w86] -> w71
        stop <- w86 stop-if-true
        n72 = Dequeue Element(queue=w91) -> (queue out=w90:refnum<queue>, element=w92:string, error out=w93:errorcluster)  [unwired: 2 in, 1 out]
        n73 = case shown="No Error" w93 {
          selector: w93 -> [w98 _]
          tunnel: w92 -> [w100 _]
          tunnel: [w94 TRUE] -> w86
          tunnel: w90 -> [w99 _]
          tunnel: w89 -> [w97 _]
          tunnel: w88 -> [w96 _]
          tunnel: w87 -> [w95 _]
          frame No Error {
            n74 = case shown="\"VNA LOOP\", Default" w100 {
              selector: w100 -> [w107 w170 w414 _ w512 w517 w539 _ w712]
              tunnel: w99 -> [w105 w166 _ _ _ _ _ _ _]
              tunnel: w98 -> [_ _ _ _ _ _ _ _ _]
              tunnel: w97 -> [w104 w168 w412 _ _ w516 _ _ w715]
              tunnel: w96 -> [w103 _ _ _ _ _ _ _ _]
              tunnel: w95 -> [w102 w167 w411 _ _ w515 _ _ w714]
              tunnel: [FALSE FALSE FALSE FALSE FALSE FALSE FALSE FALSE TRUE] -> w94
              frame "VNA LOOP", Default {
                n75 = local write "STATUS"(w107) -> ()
                n76 = stacked-sequence {
                  tunnel: w104 -> [w112 _ _]
                  tunnel: w103 -> [_ _ _]
                  tunnel: w102 -> [w111 _ _]
                  tunnel: w105 -> [_ _ w162]
                  frame #0 {
                    n77 = local read "BTN AVG ENABLE"() -> (w116:bool)
                    n78 = local read "AVG Nb"() -> (w114:i32)
                    n79 = Select(t=w114, s=w116, f=1) -> (s? t:f=w115:i32)
                    n80 = local read "SPECTRUM POST PROCESSING PARAMETERS"() -> (w122:cluster{"N° SMOOTHING POINTS":i32})
                    n81 = Unbundle By Name(w122) -> ("N° SMOOTHING POINTS"=w121:i32)
                    n82 = for {
                      N: w115 -> [_]
                      tunnel: w112 -> [w139]
                      tunnel: w111 -> [w138]
                      tunnel: w121 -> [w130]
                      tunnel: [w129] -> w118 mode=indexing
                      i -> [w127]
                      n83 = local read "RP VNA SETTING"() -> (w134:T1)
                      n84 = Increment(x=w127) -> (x+1=w126:i32)
                      n85 = local write "AVG Curr"(w126) -> ()
                      n86 = local read "BTN MAG/VEL"() -> (w128:bool)
                      n87 = local read "RAW Freq table"() -> (w131:dbl[])
                      n88 = local read "DARK SUB ?"() -> (w125:bool)
                      n89 = Unbundle By Name(w134) -> ("Sweep size"=w133:u32)
                      n90 = call "VNARP-CASES.vi"("entrée d'erreur (pas d'erreur)"=w138, "Setting"=u32 0, "Énum"=T10."SWEEP START", "ID de connexion"=w139) -> ("sortie d'erreur"=w132:errorcluster, "ID de connexion en sortie"=w135:refnum<k5>)  [unwired: 3 in]
                      n91 = call "VNARP-Read.vi"("DARK SUB ?"=w125, "SIZE"=w133, "MAG/VELOCITY"=w128, "entrée d'erreur (pas d'erreur)"=w132, "smoothing points"=w130, "Freq table IN"=w131, "ID de connexion"=w135) -> ("DATA OUT"=w129:T12)  [unwired: 2 in, 2 out]
                    }
                    n92 = call "220613 VNA DATA TO AVG.vi"("Array of SD to average"=w118) -> ("AVERAGED SD"=w117:T12)  [unwired: 2 in]
                    n93 = Unbundle By Name(w117) -> ("FREQUENCY"=w120:sgl[], "MAGNITUDE 1"=w119:dbl[], "PHASE 1"=w108:dbl[], "REAL 1"=w109:dbl[], "IMAGINARY 1"=w110:sgl[])
                    n94 = local read "VNA DATA CLUSTER"() -> (w124:T9)
                    n95 = Bundle By Name(cluster=w124, "FREQUENCY TABLE"=w120, "MAGNITUDE TABLE"=w119, "PHASE TABLE"=w108, "REAL TABLE"=w109, "IMAGINARY TABLE"=w110) -> (w123:T9)
                    n96 = local write "VNA DATA CLUSTER"(w123) -> ()
                  }
                  frame #1 {
                    n97 = local read "PERSISTANCE DATA CLUSTER"() -> (w147:T9)
                    n98 = local read "VNA DATA CLUSTER"() -> (w144:T9)
                    n99 = local read "BTN VIEW PERSISTANCE"() -> (w146:bool)
                    n100 = local read "BTN DISPLAY TYPE"() -> (w148:bool)
                    n101 = local read "RP VNA SETTING"() -> (w145:T1)
                    n102 = local read "RESONNANCE DETECTION"() -> (w143:T6)
                    n103 = call "MAKE DISPLAY ARRAY.vi"("VNA DATA CLUSTER"=w144, "PERSISTANCE DATA CLUSTER"=w147, "Display type (F : MAG/PHASE)"=w148, "Persistance"=w146) -> ("Display array"=w141:T13)  [unwired: 2 in]
                    n104 = local read "BTN FIT DISPLAY"() -> (w142:bool)
                    n105 = case shown="True" w142 {
                      tunnel: w143 -> [_ w157]
                      tunnel: w144 -> [_ w154]
                      tunnel: w145 -> [_ w153]
                      tunnel: w141 -> [w149 w151]
                      tunnel: [w149 w150] -> w140
                      frame False {
                      }
                      frame True {
                        n106 = Bundle By Name(cluster=w157, "METHOD"=u16 1) -> (w155:T6)
                        n107 = call "VNARP-Detect resonance.vi"("RP VNA SETTING"=w153, "VNA DATA CLUSTER"=w154, "RESONNANCE DETECTION"=w155) -> ("Parabolic fit"=w152:cluster{cluster{dbl, dbl}[]})  [unwired: 6 in, 2 out]
                        n108 = Insert Into Array(array=w151, new element=w152) -> (w150:T13)  [unwired: 1 in]
                      }
                    }
                    n109 = property on="MAGNITUDE/PHASE" class="XYGraph (strict)"("Val(Sgnl)"=w140) -> ()  [unwired: 2 in, 2 out]
                  }
                  frame #2 {
                    n110 = local read "LOOP ACT"() -> (w161:bool)
                    n111 = Select(t="VNA LOOP" ("element"), s=w161, f="WAIT" ("element")) -> (s? t:f=w160:string)
                    n112 = Enqueue Element(queue=w162, element=w160) -> ()  [unwired: 2 in, 3 out]
                    n113 = stacked-sequence {
                      frame #0 {
                        n114 = local write "ACQ Indicator"(TRUE ("ACQ Indicator")) -> ()
                      }
                      frame #1 {
                        n115 = Wait (ms)(milliseconds to wait=u32 100 ("attente (ms)")) -> ()  [unwired: 1 out]
                      }
                      frame #2 {
                        n116 = local write "ACQ Indicator"(FALSE ("ACQ Indicator")) -> ()
                      }
                    }
                  }
                }
                n117 = Wait (ms)(milliseconds to wait=u32 10 ("attente (ms)")) -> ()  [unwired: 1 out]
              }
              frame "TRACK" {
                n118 = local write "STATUS"(w170) -> ()
                n119 = stacked-sequence {
                  tunnel: w168 -> [_ w177 _]
                  tunnel: w167 -> [_ w176 _]
                  tunnel: w166 -> [_ w175 w406]
                  frame #0 {
                    n120 = local read "DELAY BETWEEN TRIG (s)"() -> (w173:i32)
                    n121 = Multiply(x=w173, y=u32 1000 ("attente (ms)")) -> (x*y=w172:u32)
                    n122 = Wait (ms)(milliseconds to wait=w172) -> ()  [unwired: 1 out]
                  }
                  frame #1 {
                    n123 = local read "CHANNELS PARAMETERS"() -> (w174:T4[])
                    n124 = for {
                      tunnel: w174 -> [w183] mode=indexing
                      tunnel: w177 -> [w182]
                      tunnel: w176 -> [w181]
                      tunnel: w175 -> [w179]
                      tunnel: w174 -> [w178]
                      i -> [w180]
                      n125 = Unbundle By Name(w183) -> ("CHANNEL TRACK ?"=w184:bool)
                      n126 = case shown="True" w184 {
                        tunnel: w183 -> [_ w186]
                        tunnel: w182 -> [_ w187]
                        tunnel: w181 -> [_ w189]
                        tunnel: w180 -> [_ w188]
                        tunnel: w179 -> [_ _]
                        tunnel: w178 -> [_ w185]
                        frame False {
                        }
                        frame True {
                          n127 = stacked-sequence {
                            tunnel: w189 -> [_ w203 _ _ _ w237 w251 _ _ _ _ _ _ _ _]
                            tunnel: w188 -> [w190 _ w208 _ w228 _ _ _ w292 w297 w316 _ _ _ _]
                            tunnel: w187 -> [_ w194 _ _ _ w234 w252 _ _ _ _ _ _ _ _]
                            tunnel: w186 -> [_ w193 _ _ w229 _ _ _ _ _ _ _ _ _ _]
                            tunnel: w185 -> [_ _ _ _ w227 _ _ _ _ _ _ _ _ _ _]
                            frame #0 {
                              # "ATTENTION : do not trig channel choice change event !!!!"
                              # "switch"
                              n128 = local write "CHANNEL CHOICE VNA"(w190) -> ()
                              n129 = local write "CHANNELS IND TRACK"(w190) -> ()
                            }
                            frame #1 {
                              n130 = local write "VNA SETTING CLUSTER"(w193) -> ()
                              n131 = local read "RP VNA SETTING"() -> (w206:T1)
                              n132 = call "VNARP-VNASETTING CLTR MANAGMENT.vi"("VNA SETTING CLUSTER"=w193, "RP VNA SETTING"=w206) -> ("OUTPUT VNA SETTINGS"=w204:T14)  [unwired: 1 in]
                              n133 = local write "RP VNA SETTING"(w204) -> ()
                              n134 = call "VNARP-SettingsUpdate.vi"("Error IN"=w203, "RP VNA SETTINGS IN"=w204, "ID de connexion IN"=w194) -> ("Freq table"=w205:dbl[])  [unwired: 2 out]
                              n135 = local write "RAW Freq table"(w205) -> ()
                              n136 = Unbundle By Name(w193) -> ("START 2"=w196:dbl, "STOP 2"=w202:dbl, "CENTER 2"=w201:dbl, "SPAN 2"=w200:dbl, "PUMP"=w195:dbl, "PROBE"=w199:dbl, "Points N° 2"=w198:i32, "SPACING 2"=w197:dbl, "AVG"=w192:i32, "AVG ENABLE"=w191:bool)
                              n137 = local write "BTN AVG ENABLE"(w191) -> ()
                              n138 = local write "AVG Nb"(w192) -> ()
                              n139 = local write "SPACING"(w197) -> ()
                              n140 = local write "Points N°"(w198) -> ()
                              n141 = local write "CENTER"(w201) -> ()
                              n142 = local write "START"(w196) -> ()
                              n143 = local write "STOP"(w202) -> ()
                              n144 = local write "PROBE"(w199) -> ()
                              n145 = local write "SPAN"(w200) -> ()
                              n146 = local write "PUMP"(w195) -> ()
                              n147 = property on="START" class="DigNum (strict)"("Val(Sgnl)"=w196) -> ()  [unwired: 2 in, 2 out]
                              n148 = property on="PUMP" class="Slide (strict)"("Val(Sgnl)"=w195) -> ()  [unwired: 2 in, 2 out]
                            }
                            frame #2 {
                              w219 = u16 0 items=["AOUT0", "AOUT1", "AOUT2", "AOUT3"] ("Pin #")
                              w218 = u16 1 items=["AOUT0", "AOUT1", "AOUT2", "AOUT3"] ("Pin #")
                              n149 = local read "NETWORK PARAMETERS"() -> (w220:T8)
                              n150 = local read "VOA Calibration cluster"() -> (w217:cluster{"PUMP":dbl[], "PROBE":dbl[]})
                              n151 = Unbundle By Name(w220) -> ("RP-IP 2"=w209:string)
                              n152 = Unbundle By Name(w217) -> ("PUMP"=w212:dbl[], "PROBE"=w215:dbl[])
                              n153 = local read "PUMP"() -> (w213:dbl)
                              n154 = local read "PROBE"() -> (w216:dbl)
                              n155 = call "RP-VOA CONVERSION P to V.vi"("Calibration points"=w212, "% power"=w213) -> ("DAC Voltage"=w211:dbl)
                              n156 = call "RP-VOA CONVERSION P to V.vi"("Calibration points"=w215, "% power"=w216) -> ("DAC Voltage"=w214:dbl)
                              n157 = local read "Enable optical switch"() -> (w207:bool)
                              n158 = Increment(x=w208) -> (x+1=w210:i32)
                              n159 = case shown="True" w207 {
                                tunnel: w210 -> [_ w222]
                                tunnel: w209 -> [_ w221]
                                frame False {
                                }
                                frame True {
                                n160 = call "RP-SWITCH CHANNEL.vi"("Channel"=w222, "IP address"=w221) -> ()  [unwired: 1 in, 2 out]
                                }
                              }
                              n161 = call "RP-ANALOG-OUT.vi"("Voltage"=w211, "Pin #"=w219, "IP address"=w209) -> ()  [unwired: 1 out]
                              n162 = call "RP-ANALOG-OUT.vi"("Voltage"=w214, "Pin #"=w218, "IP address"=w209) -> ()  [unwired: 1 out]
                            }
                            frame #3 {
                              n163 = local read "VNA SETTING CLUSTER"() -> (w226:T4)
                              n164 = local read "PROBE"() -> (w224:dbl)
                              n165 = local read "PUMP"() -> (w225:dbl)
                              n166 = Bundle By Name(cluster=w226, "PUMP"=w225, "PROBE"=w224) -> (w223:T4)
                              n167 = local write "VNA SETTING CLUSTER"(w223) -> ()
                            }
                            frame #4 {
                              n168 = local read "VNA SETTING CLUSTER"() -> (w232:T4)
                              n169 = Unbundle By Name(w229) -> ("CHANNEL TRACK ?"=w231:bool)
                              n170 = Bundle By Name(cluster=w232, "CHANNEL TRACK ?"=w231) -> (w230:T4)
                              n171 = Replace Array Subset(array=w227, new element=w230, index=w228) -> (w233:T4[])
                              n172 = local write "CHANNELS PARAMETERS"(w233) -> ()
                            }
                            frame #5 {
                              # "wait for stab"
                              n173 = local read "DELAY AFTER SWITCH (s)"() -> (w236:i32)
                              n174 = Equal To 0?(x=w236) -> (x = 0?=w235:bool)
                              n175 = case shown="False" w235 {
                                tunnel: w237 -> [w239 _]
                                tunnel: w234 -> [w238 _]
                                frame False {
                                n176 = Tick Count (ms)() -> (millisecond timer value=w240:u32)
                                n177 = while {
                                tunnel: w240 -> [w249]
                                tunnel: w239 -> [w243]
                                tunnel: w238 -> [w242]
                                stop <- w244 stop-if-true
                                n178 = flat-sequence {
                                tunnel: w243 -> [_]
                                tunnel: w242 -> [_]
                                tunnel: [w250] -> w241
                                frame #0 {
                                }
                                frame #1 {
                                n179 = Tick Count (ms)() -> (millisecond timer value=w250:u32)
                                }
                                }
                                n180 = local read "DELAY AFTER SWITCH (s)"() -> (w248:i32)
                                n181 = Subtract(x=w241, y=w249) -> (x-y=w246:u32)
                                n182 = Multiply(x=w248, y=1000) -> (x*y=w245:i32)
                                n183 = Greater Or Equal?(x=w246, y=w245) -> (x >= y?=w244:bool)
                                }
                                }
                                frame True {
                                }
                              }
                            }
                            frame #6 {
                              n184 = local read "BTN AVG ENABLE"() -> (w256:bool)
                              n185 = local read "AVG Nb"() -> (w254:i32)
                              n186 = local read "SPECTRUM POST PROCESSING PARAMETERS"() -> (w265:cluster{"N° SMOOTHING POINTS":i32})
                              n187 = Select(t=w254, s=w256, f=1) -> (s? t:f=w255:i32)
                              n188 = Unbundle By Name(w265) -> ("N° SMOOTHING POINTS"=w264:i32)
                              n189 = for {
                                N: w255 -> [_]
                                tunnel: w252 -> [w283]
                                tunnel: w251 -> [w282]
                                tunnel: w264 -> [w274]
                                tunnel: [w273] -> w258 mode=indexing
                                i -> [w271]
                                n190 = local read "RP VNA SETTING"() -> (w278:T1)
                                n191 = Increment(x=w271) -> (x+1=w270:i32)
                                n192 = local read "BTN MAG/VEL"() -> (w272:bool)
                                n193 = local read "RAW Freq table"() -> (w275:dbl[])
                                n194 = local write "AVG Curr"(w270) -> ()
                                n195 = Unbundle By Name(w278) -> ("Sweep size"=w277:u32)
                                n196 = local read "DARK SUB ?"() -> (w269:bool)
                                n197 = call "VNARP-CASES.vi"("entrée d'erreur (pas d'erreur)"=w282, "Setting"=u32 0, "Énum"=T10."SWEEP START", "ID de connexion"=w283) -> ("sortie d'erreur"=w276:errorcluster, "ID de connexion en sortie"=w279:refnum<k5>)  [unwired: 3 in]
                                n198 = call "VNARP-Read.vi"("DARK SUB ?"=w269, "SIZE"=w277, "MAG/VELOCITY"=w272, "entrée d'erreur (pas d'erreur)"=w276, "smoothing points"=w274, "Freq table IN"=w275, "ID de connexion"=w279) -> ("DATA OUT"=w273:T12)  [unwired: 2 in, 2 out]
                              }
                              n199 = call "220613 VNA DATA TO AVG.vi"("Array of SD to average"=w258) -> ("AVERAGED SD"=w257:T12)  [unwired: 2 in]
                              n200 = local read "CHANNEL CHOICE VNA"() -> (w268:T3)
                              n201 = Unbundle By Name(w257) -> ("FREQUENCY"=w263:sgl[], "MAGNITUDE 1"=w262:dbl[], "PHASE 1"=w261:dbl[], "REAL 1"=w260:dbl[], "IMAGINARY 1"=w259:sgl[])
                              n202 = local read "VNA DATA CLUSTER"() -> (w267:T9)
                              n203 = Bundle By Name(cluster=w267, "CHANNEL"=w268, "FREQUENCY TABLE"=w263, "MAGNITUDE TABLE"=w262, "PHASE TABLE"=w261, "REAL TABLE"=w260, "IMAGINARY TABLE"=w259) -> (w266:T9)
                              n204 = local write "VNA DATA CLUSTER"(w266) -> ()
                            }
                            frame #7 {
                              n205 = local read "PERSISTANCE DATA CLUSTER"() -> (w286:T9)
                              n206 = local read "VNA DATA CLUSTER"() -> (w287:T9)
                              n207 = local read "BTN DISPLAY TYPE"() -> (w288:bool)
                              n208 = local read "BTN VIEW PERSISTANCE"() -> (w285:bool)
                              n209 = call "MAKE DISPLAY ARRAY.vi"("VNA DATA CLUSTER"=w287, "PERSISTANCE DATA CLUSTER"=w286, "Display type (F : MAG/PHASE)"=w288, "Persistance"=w285) -> ("Display array"=w284:T13)  [unwired: 2 in]
                              n210 = local write "MAGNITUDE/PHASE"(w284) -> ()
                              n211 = property on="MAGNITUDE/PHASE" class="XYGraph (strict)"("Val(Sgnl)"=w284) -> ()  [unwired: 2 in, 2 out]
                              n212 = stacked-sequence {
                                frame #0 {
                                n213 = local write "ACQ Indicator"(TRUE ("ACQ Indicator")) -> ()
                                }
                                frame #1 {
                                n214 = Wait (ms)(milliseconds to wait=u32 100) -> ()  [unwired: 1 out]
                                }
                                frame #2 {
                                n215 = local write "ACQ Indicator"(FALSE ("ACQ Indicator")) -> ()
                                }
                              }
                            }
                            frame #8 {
                              n216 = local read "VNA DATA CLUSTER TBL"() -> (w294:T9[])
                              n217 = local read "VNA DATA CLUSTER"() -> (w293:T9)
                              n218 = Replace Array Subset(array=w294, new element=w293, index=w292) -> (w295:T9[])
                              n219 = local write "VNA DATA CLUSTER TBL"(w295) -> ()
                            }
                            frame #9 {
                              n220 = local read "BTN AUTOSAVE RAW DATA"() -> (w296:bool)
                              n221 = case shown="True" w296 {
                                tunnel: w297 -> [_ w299]
                                frame False {
                                }
                                frame True {
                                # "save to file vna"
                                n222 = local read "VNA DATA CLUSTER TBL"() -> (w310:T9[])
                                n223 = local read "Track Repositery List"() -> (w300:path[])
                                n224 = Tick Count (ms)() -> (millisecond timer value=w308:u32)
                                n225 = Number To Decimal String(number=w308) -> (decimal integer string=w307:string)  [unwired: 1 in]
                                n226 = call "RP-VNA DATA TBL Extract.vi"("VNA DATA CLUSTER TBL"=w310, "index"=w299) -> ("appended array"=w309:ext[][])  [unwired: 2 in, 1 out]
                                n227 = Concatenate Strings("RAW VNA DATA " ("string"), w307, ".txt" ("string")) -> (w305:string)
                                n228 = Index Array(array=w300, index=w299) -> (element=w298:path)
                                n229 = Build Path(base path=w298, name or relative path=w305) -> (appended path=w304:path)
                                n230 = call-poly <vilib>:"Write Delimited Spreadsheet.vi"("file path (dialog if empty)"=w304, "format (%.3f)"="%.6f", "2D data"=w309, "transpose? (no:F)"=TRUE) -> ()  [unwired: 10 in, 2 out]
                                }
                              }
                            }
                            frame #10 {
                              # "add to track kpi tables"
                              n231 = local read "RESONNANCE DETECTION"() -> (w313:T6)
                              n232 = local read "VNA DATA CLUSTER"() -> (w312:T9)
                              n233 = local read "RP VNA SETTING"() -> (w311:T1)
                              n234 = local read "TRACK DATA CLUSTER TBL"() -> (w318:cluster{"CHANNEL":dbl, "KPI 1 TRACK":ext[]}[])
                              n235 = local read "BTN FIT DISPLAY"() -> (w314:bool)
                              n236 = call "VNARP-Detect resonance.vi"("RP VNA SETTING"=w311, "VNA DATA CLUSTER"=w312, "RESONNANCE DETECTION"=w313) -> ("Resonant frequency"=w315:ext)  [unwired: 6 in, 2 out]
                              n237 = Index Array(array=w318, index=w316) -> (element=w320:cluster{"CHANNEL":dbl, "KPI 1 TRACK":ext[]})
                              n238 = Unbundle By Name(w320) -> ("KPI 1 TRACK"=w322:ext[])
                              n239 = case shown="True" w314 {
                                tunnel: w313 -> [_ w328]
                                tunnel: w312 -> [_ w325]
                                tunnel: w311 -> [_ w324]
                                frame False {
                                }
                                frame True {
                                n240 = Bundle By Name(cluster=w328, "METHOD"=u16 1) -> (w326:T6)
                                n241 = property on="MAGNITUDE/PHASE" class="XYGraph (strict)"() -> ("Value"=w330:cluster{cluster{dbl, dbl}[]}[])  [unwired: 2 in, 2 out]
                                n242 = call "VNARP-Detect resonance.vi"("RP VNA SETTING"=w324, "VNA DATA CLUSTER"=w325, "RESONNANCE DETECTION"=w326) -> ("Parabolic fit"=w323:cluster{cluster{dbl, dbl}[]})  [unwired: 6 in, 2 out]
                                n243 = Insert Into Array(array=w330, new element=w323) -> (w329:cluster{cluster{dbl, dbl}[]}[])  [unwired: 1 in]
                                n244 = property on="MAGNITUDE/PHASE" class="XYGraph (strict)"("Val(Sgnl)"=w329) -> ()  [unwired: 2 in, 2 out]
                                }
                              }
                              n245 = Build Array (concatenate)(w322, w315) -> (w321:ext[])
                              n246 = Bundle By Name(cluster=w320, "CHANNEL"=w316, "KPI 1 TRACK"=w321) -> (w319:cluster{"CHANNEL":dbl, "KPI 1 TRACK":ext[]})
                              n247 = Replace Array Subset(array=w318, new element=w319, index=w316) -> (w317:cluster{"CHANNEL":dbl, "KPI 1 TRACK":ext[]}[])
                              n248 = local write "TRACK DATA CLUSTER TBL"(w317) -> ()
                            }
                            frame #11 {
                              n249 = local read "TRACK DATA CLUSTER TBL"() -> (w334:cluster{"CHANNEL":dbl, "KPI 1 TRACK":ext[]}[])
                              n250 = for {
                                tunnel: w334 -> [w359] mode=indexing
                                tunnel: [w337] -> w333 mode=indexing
                                tunnel: [w336] -> w332 mode=indexing
                                tunnel: [w335] -> w331 mode=indexing
                                n251 = local read "TEMPORAL SMOOTHING"() -> (w356:i32)
                                n252 = Unbundle By Name(w359) -> ("KPI 1 TRACK"=w355:ext[])
                                n253 = Array Size(array=w355) -> (size(s)=w357:i32)
                                n254 = Subtract(x=w357, y=w356) -> (x-y=w358:i32)
                                n255 = for {
                                N: w358 -> [_]
                                tunnel: w356 -> [w363]
                                tunnel: w355 -> [w364]
                                tunnel: [w360] -> w344 mode=indexing
                                i -> [w362]
                                n256 = Array Subset(array=w364, index=w362, length=w363) -> (w361:ext[])
                                n257 = call-poly <vilib>:"Mean.vi"("X"=w361) -> ("mean"=w360:dbl)  [unwired: 1 out]
                                }
                                n258 = Delete From Array(array=w344, length=1, index=0) -> (array with subset deleted=w336:dbl[])  [unwired: 1 out]
                                n259 = local read "DISPLAY OPTION"() -> (w353:u16)
                                n260 = Index Array(array=w336, index=0) -> (element=w348:dbl)
                                n261 = local read "N°POINTS TO DISPLAY"() -> (w340:i32)
                                n262 = Subtract(x=w336, y=w348) -> (x-y=w349:dbl[])
                                n263 = Divide(x=w349, y=w348) -> (x/y=w347:dbl[])
                                n264 = Equal?(x=w353, y=u16 0) -> (x = y?=w345:bool)
                                n265 = Multiply(x=w347, y=1000000.0 ("f")) -> (x*y=w335:dbl[])
                                n266 = Select(t=w336, s=w345, f=w335) -> (s? t:f=w338:dbl[])
                                n267 = Array Size(array=w338) -> (size(s)=w342:i32)
                                n268 = Subtract(x=w342, y=w340) -> (x-y=w341:i32)
                                n269 = Max & Min(x=0.0, y=w341) -> (max(x,y)=w343:dbl)  [unwired: 1 out]
                                n270 = Array Subset(array=w338, index=w343) -> (w337:dbl[])  [unwired: 1 in]
                              }
                              n271 = local write "TRACK DATA ABS"(w332) -> ()
                              n272 = local write "TRACK DATA REL"(w331) -> ()
                              n273 = local write "LIVE TRACK"(w333) -> ()
                            }
                            frame #12 {
                              n274 = local read "TRACK DATA CLUSTER TBL"() -> (w367:cluster{"CHANNEL":dbl, "KPI 1 TRACK":ext[]}[])
                              n275 = for {
                                tunnel: w367 -> [w380] mode=indexing
                                tunnel: [w371] -> w366 mode=indexing
                                tunnel: [w370] -> w365 mode=indexing
                                n276 = Unbundle By Name(w380) -> ("KPI 1 TRACK"=w369:ext[])
                                n277 = local read "DISPLAY OPTION"() -> (w378:u16)
                                n278 = Delete From Array(array=w369, length=1, index=0) -> (array with subset deleted=w371:ext[])  [unwired: 1 out]
                                n279 = Equal?(x=w378, y=u16 0) -> ()  [unwired: 1 out]
                                n280 = Index Array(array=w371, index=0) -> (element=w373:ext)
                                n281 = Subtract(x=w371, y=w373) -> (x-y=w374:ext[])
                                n282 = Divide(x=w374, y=w373) -> (x/y=w372:ext[])
                                n283 = Multiply(x=w372, y=1000000.0 ("f")) -> (x*y=w370:ext[])
                              }
                              n284 = local write "TRACK DATA ABS NO SMOOTHING"(w366) -> ()
                              n285 = local write "TRACK DATA REL NO SMOOTHING"(w365) -> ()
                            }
                            frame #13 {
                              n286 = local read "TRACK DATA ABS NO SMOOTHING"() -> (w389:dbl[][])
                              n287 = local read "TRACK REPOSITERY"() -> (w402:path)
                              n288 = local read "TRACK REPOSITERY"() -> (w383:path)
                              n289 = local read "TRACK DATA ABS"() -> (w396:dbl[][])
                              n290 = Build Path(base path=w402, name or relative path="ALL CHANNEL ABS Track.txt") -> (appended path=w403:path)
                              n291 = Build Path(base path=w383, name or relative path="ALL CHANNEL ABS Track NS.txt") -> (appended path=w382:path)
                              n292 = call-poly <vilib>:"Write Delimited Spreadsheet.vi"("file path (dialog if empty)"=w403, "format (%.3f)"="%.6f", "2D data"=w396, "transpose? (no:F)"=TRUE) -> ()  [unwired: 10 in, 2 out]
                              n293 = call-poly <vilib>:"Write Delimited Spreadsheet.vi"("file path (dialog if empty)"=w382, "format (%.3f)"="%.6f", "2D data"=w389, "transpose? (no:F)"=TRUE) -> ()  [unwired: 10 in, 2 out]
                              n294 = local read "TRACK DATA REL NO SMOOTHING"() -> (w390:dbl[][])
                              n295 = local read "TRACK REPOSITERY"() -> (w399:path)
                              n296 = local read "TRACK REPOSITERY"() -> (w386:path)
                              n297 = local read "TRACK DATA REL"() -> (w395:dbl[][])
                              n298 = Build Path(base path=w399, name or relative path="ALL CHANNEL REL Track.txt") -> (appended path=w398:path)
                              n299 = Build Path(base path=w386, name or relative path="ALL CHANNEL REL Track NS.txt") -> (appended path=w387:path)
                              n300 = call-poly <vilib>:"Write Delimited Spreadsheet.vi"("file path (dialog if empty)"=w398, "format (%.3f)"="%.6f", "2D data"=w395, "transpose? (no:F)"=TRUE) -> ()  [unwired: 10 in, 2 out]
                              n301 = call-poly <vilib>:"Write Delimited Spreadsheet.vi"("file path (dialog if empty)"=w387, "format (%.3f)"="%.6f", "2D data"=w390, "transpose? (no:F)"=TRUE) -> ()  [unwired: 10 in, 2 out]
                            }
                            frame #14 {
                            }
                          }
                        }
                      }
                    }
                  }
                  frame #2 {
                    n302 = local read "LOOP ACT"() -> (w409:bool)
                    n303 = Select(t="TRACK" ("element"), s=w409, f="WAIT" ("element")) -> (s? t:f=w408:string)
                    n304 = Enqueue Element(queue=w406, element=w408) -> ()  [unwired: 2 in, 3 out]
                  }
                }
              }
              frame "RUN VNA" {
                n305 = local write "STATUS"(w414) -> ()
                n306 = stacked-sequence {
                  tunnel: w412 -> [w431 _ _]
                  tunnel: w411 -> [w430 _ _]
                  frame #0 {
                    n307 = local read "BTN AVG ENABLE"() -> (w418:bool)
                    n308 = local read "AVG Nb"() -> (w415:i32)
                    n309 = Select(t=w415, s=w418, f=1) -> (s? t:f=w417:i32)
                    n310 = local read "SPECTRUM POST PROCESSING PARAMETERS"() -> (w427:cluster{"N° SMOOTHING POINTS":i32})
                    n311 = Unbundle By Name(w427) -> ("N° SMOOTHING POINTS"=w426:i32)
                    n312 = for {
                      N: w417 -> [_]
                      tunnel: w431 -> [w446]
                      tunnel: w430 -> [w445]
                      tunnel: w426 -> [w437]
                      tunnel: [w436] -> w420 mode=indexing
                      i -> [w434]
                      n313 = local read "RP VNA SETTING"() -> (w441:T1)
                      n314 = Increment(x=w434) -> (x+1=w433:i32)
                      n315 = local write "AVG Curr"(w433) -> ()
                      n316 = local read "BTN MAG/VEL"() -> (w435:bool)
                      n317 = local read "RAW Freq table"() -> (w438:dbl[])
                      n318 = Unbundle By Name(w441) -> ("Sweep size"=w440:u32)
                      n319 = local read "DARK SUB ?"() -> (w432:bool)
                      n320 = call "VNARP-CASES.vi"("entrée d'erreur (pas d'erreur)"=w445, "Setting"=u32 0, "Énum"=T10."SWEEP START", "ID de connexion"=w446) -> ("sortie d'erreur"=w439:errorcluster, "ID de connexion en sortie"=w442:refnum<k5>)  [unwired: 3 in]
                      n321 = call "VNARP-Read.vi"("DARK SUB ?"=w432, "SIZE"=w440, "MAG/VELOCITY"=w435, "entrée d'erreur (pas d'erreur)"=w439, "smoothing points"=w437, "Freq table IN"=w438, "ID de connexion"=w442) -> ("DATA OUT"=w436:T12)  [unwired: 2 in, 2 out]
                    }
                    n322 = call "220613 VNA DATA TO AVG.vi"("Array of SD to average"=w420) -> ("AVERAGED SD"=w419:T12)  [unwired: 2 in]
                    n323 = Unbundle By Name(w419) -> ("FREQUENCY"=w425:sgl[], "MAGNITUDE 1"=w424:dbl[], "PHASE 1"=w423:dbl[], "REAL 1"=w422:dbl[], "IMAGINARY 1"=w421:sgl[])
                    n324 = local read "VNA DATA CLUSTER"() -> (w429:T9)
                    n325 = Bundle By Name(cluster=w429, "FREQUENCY TABLE"=w425, "MAGNITUDE TABLE"=w424, "PHASE TABLE"=w423, "REAL TABLE"=w422, "IMAGINARY TABLE"=w421) -> (w428:T9)
                    n326 = local write "VNA DATA CLUSTER"(w428) -> ()
                  }
                  frame #1 {
                    n327 = local read "VNA DATA CLUSTER"() -> (w451:T9)
                    n328 = local read "PERSISTANCE DATA CLUSTER"() -> (w454:T9)
                    n329 = local read "BTN DISPLAY TYPE"() -> (w455:bool)
                    n330 = local read "BTN VIEW PERSISTANCE"() -> (w453:bool)
                    n331 = local read "RESONNANCE DETECTION"() -> (w448:T6)
                    n332 = local read "RP VNA SETTING"() -> (w449:T1)
                    n333 = local read "BTN FIT DISPLAY"() -> (w450:bool)
                    n334 = call "MAKE DISPLAY ARRAY.vi"("VNA DATA CLUSTER"=w451, "PERSISTANCE DATA CLUSTER"=w454, "Display type (F : MAG/PHASE)"=w455, "Persistance"=w453) -> ("Display array"=w452:T13)  [unwired: 2 in]
                    n335 = case shown="True" w450 {
                      tunnel: w448 -> [_ w464]
                      tunnel: w451 -> [_ w461]
                      tunnel: w449 -> [_ w460]
                      tunnel: w452 -> [w456 w458]
                      tunnel: [w456 w457] -> w447
                      frame False {
                      }
                      frame True {
                        n336 = Bundle By Name(cluster=w464, "METHOD"=u16 1) -> (w462:T6)
                        n337 = call "VNARP-Detect resonance.vi"("RP VNA SETTING"=w460, "VNA DATA CLUSTER"=w461, "RESONNANCE DETECTION"=w462) -> ("Parabolic fit"=w459:cluster{cluster{dbl, dbl}[]})  [unwired: 6 in, 2 out]
                        n338 = Insert Into Array(array=w458, new element=w459) -> (w457:T13)  [unwired: 1 in]
                      }
                    }
                    n339 = property on="MAGNITUDE/PHASE" class="XYGraph (strict)"("Val(Sgnl)"=w447) -> ()  [unwired: 2 in, 2 out]
                  }
                  frame #2 {
                    n340 = stacked-sequence {
                      frame #0 {
                        n341 = local write "ACQ Indicator"(TRUE ("ACQ Indicator")) -> ()
                      }
                      frame #1 {
                        n342 = Wait (ms)(milliseconds to wait=u32 100 ("attente (ms)")) -> ()  [unwired: 1 out]
                      }
                      frame #2 {
                        n343 = local write "ACQ Indicator"(FALSE ("ACQ Indicator")) -> ()
                      }
                    }
                  }
                }
                n344 = Wait (ms)(milliseconds to wait=u32 10 ("attente (ms)")) -> ()  [unwired: 1 out]
              }
              frame "CHANNEL CHANGE" {
                n345 = stacked-sequence {
                  frame #0 {
                    n346 = local read "CHANNEL CHOICE VNA"() -> (w482:T3)
                    n347 = local read "CHANNELS PARAMETERS"() -> (w483:T4[])
                    n348 = Index Array(array=w483, index=w482) -> (element=w479:T4)
                    n349 = local write "VNA SETTING CLUSTER"(w479) -> ()
                    n350 = local read "RP VNA SETTING"() -> (w480:T1)
                    n351 = Unbundle By Name(w479) -> ("START 2"=w473:dbl, "STOP 2"=w478:dbl, "CENTER 2"=w477:dbl, "SPAN 2"=w476:dbl, "PUMP"=w471:dbl, "PROBE"=w472:dbl, "Points N° 2"=w475:i32, "SPACING 2"=w474:dbl, "AVG"=w470:i32, "AVG ENABLE"=w469:bool)
                    n352 = local write "Points N°"(w475) -> ()
                    n353 = local write "BTN AVG ENABLE"(w469) -> ()
                    n354 = local write "AVG Nb"(w470) -> ()
                    n355 = local write "CENTER"(w477) -> ()
                    n356 = local write "SPACING"(w474) -> ()
                    n357 = local write "START"(w473) -> ()
                    n358 = local write "STOP"(w478) -> ()
                    n359 = local write "PROBE"(w472) -> ()
                    n360 = local write "SPAN"(w476) -> ()
                    n361 = local write "PUMP"(w471) -> ()
                    n362 = call "VNARP-VNASETTING CLTR MANAGMENT.vi"("VNA SETTING CLUSTER"=w479, "RP VNA SETTING"=w480) -> ("OUTPUT VNA SETTINGS"=w481:T14)  [unwired: 1 in]
                    n363 = local write "RP VNA SETTING"(w481) -> ()
                    n364 = property on="START" class="DigNum (strict)"("Val(Sgnl)"=w473) -> ()  [unwired: 2 in, 2 out]
                  }
                  frame #1 {
                    w496 = u16 0 items=["AOUT0", "AOUT1", "AOUT2", "AOUT3"] ("Pin #")
                    w495 = u16 1 items=["AOUT0", "AOUT1", "AOUT2", "AOUT3"] ("Pin #")
                    n365 = local read "VOA Calibration cluster"() -> (w494:cluster{"PUMP":dbl[], "PROBE":dbl[]})
                    n366 = local read "NETWORK PARAMETERS"() -> (w497:T8)
                    n367 = local read "PROBE"() -> (w493:dbl)
                    n368 = Unbundle By Name(w497) -> ("RP-IP 2"=w487:string)
                    n369 = Unbundle By Name(w494) -> ("PUMP"=w488:dbl[], "PROBE"=w492:dbl[])
                    n370 = local read "PUMP"() -> (w489:dbl)
                    n371 = local read "CHANNEL CHOICE VNA"() -> (w486:T3)
                    n372 = call "RP-VOA CONVERSION P to V.vi"("Calibration points"=w488, "% power"=w489) -> ("DAC Voltage"=w490:dbl)
                    n373 = call "RP-VOA CONVERSION P to V.vi"("Calibration points"=w492, "% power"=w493) -> ("DAC Voltage"=w491:dbl)
                    n374 = local read "Enable optical switch"() -> (w484:bool)
                    n375 = Increment(x=w486) -> (x+1=w485:T3)
                    n376 = case shown="True" w484 {
                      tunnel: w487 -> [_ w499]
                      tunnel: w485 -> [_ w498]
                      frame False {
                      }
                      frame True {
                        n377 = call "RP-SWITCH CHANNEL.vi"("Channel"=w498, "IP address"=w499) -> ()  [unwired: 1 in, 2 out]
                      }
                    }
                    n378 = call "RP-ANALOG-OUT.vi"("Voltage"=w490, "Pin #"=w496, "IP address"=w487) -> ()  [unwired: 1 out]
                    n379 = call "RP-ANALOG-OUT.vi"("Voltage"=w491, "Pin #"=w495, "IP address"=w487) -> ()  [unwired: 1 out]
                  }
                  frame #2 {
                    n380 = local read "VNA SETTING CLUSTER"() -> (w503:T4)
                    n381 = local read "PROBE"() -> (w501:dbl)
                    n382 = local read "PUMP"() -> (w502:dbl)
                    n383 = Bundle By Name(cluster=w503, "PUMP"=w502, "PROBE"=w501) -> (w500:T4)
                    n384 = local write "VNA SETTING CLUSTER"(w500) -> ()
                  }
                  frame #3 {
                    n385 = local read "CHANNELS PARAMETERS"() -> (w509:T4[])
                    n386 = local read "CHANNEL CHOICE VNA"() -> (w508:T3)
                    n387 = Index Array(array=w509, index=w508) -> (element=w507:T4)
                    n388 = local read "VNA SETTING CLUSTER"() -> (w506:T4)
                    n389 = Unbundle By Name(w507) -> ("CHANNEL TRACK ?"=w505:bool)
                    n390 = Bundle By Name(cluster=w506, "CHANNEL TRACK ?"=w505) -> (w504:T4)
                    n391 = Replace Array Subset(array=w509, new element=w504, index=w508) -> (w510:T4[])
                    n392 = local write "CHANNELS PARAMETERS"(w510) -> ()
                  }
                  frame #4 {
                    n393 = local read "CHANNEL CHOICE VNA"() -> (→"CHANNEL CHOSEN":T3)
                  }
                }
              }
              frame "WAIT" {
                n394 = local write "STATUS"(w512) -> ()
              }
              frame "UPDATE" {
                n395 = local write "STATUS"(w517) -> ()
                n396 = stacked-sequence {
                  tunnel: w516 -> [w521 _ _]
                  tunnel: w515 -> [w519 _ _]
                  frame #0 {
                    n397 = local read "RP VNA SETTING"() -> (w520:T1)
                    n398 = call "VNARP-SettingsUpdate.vi"("Error IN"=w519, "RP VNA SETTINGS IN"=w520, "ID de connexion IN"=w521) -> ("Freq table"=w518:dbl[])  [unwired: 2 out]
                    n399 = local write "RAW Freq table"(w518) -> ()
                  }
                  frame #1 {
                    n400 = local read "VNA SETTING CLUSTER"() -> (w531:T4)
                    n401 = local read "BTN AVG ENABLE"() -> (w522:bool)
                    n402 = local read "Points N°"() -> (w525:i32)
                    n403 = local read "AVG Nb"() -> (w523:i32)
                    n404 = local read "SPACING"() -> (w524:dbl)
                    n405 = local read "CENTER"() -> (w527:dbl)
                    n406 = local read "START"() -> (w530:dbl)
                    n407 = local read "SPAN"() -> (w526:dbl)
                    n408 = local read "STOP"() -> (w529:dbl)
                    n409 = Bundle By Name(cluster=w531, "START 2"=w530, "STOP 2"=w529, "CENTER 2"=w527, "SPAN 2"=w526, "Points N° 2"=w525, "SPACING 2"=w524, "AVG"=w523, "AVG ENABLE"=w522) -> (w528:T4)
                    n410 = local write "VNA SETTING CLUSTER"(w528) -> ()
                  }
                  frame #2 {
                    n411 = local read "CHANNELS PARAMETERS"() -> (w537:T4[])
                    n412 = local read "CHANNEL CHOICE VNA"() -> (w536:T3)
                    n413 = Index Array(array=w537, index=w536) -> (element=w535:T4)
                    n414 = local read "VNA SETTING CLUSTER"() -> (w534:T4)
                    n415 = Unbundle By Name(w535) -> ("CHANNEL TRACK ?"=w533:bool)
                    n416 = Bundle By Name(cluster=w534, "CHANNEL TRACK ?"=w533) -> (w532:T4)
                    n417 = Replace Array Subset(array=w537, new element=w532, index=w536) -> (w538:T4[])
                    n418 = local write "CHANNELS PARAMETERS"(w538) -> ()
                  }
                }
              }
              frame "POWER UPDATE" {
                n419 = local write "STATUS"(w539) -> ()
                n420 = stacked-sequence {
                  frame #0 {
                    w549 = u16 0 items=["AOUT0", "AOUT1", "AOUT2", "AOUT3"] ("Pin #")
                    w551 = u16 1 items=["AOUT0", "AOUT1", "AOUT2", "AOUT3"] ("Pin #")
                    n421 = local read "VOA Calibration cluster"() -> (w547:cluster{"PUMP":dbl[], "PROBE":dbl[]})
                    n422 = local read "NETWORK PARAMETERS"() -> (w550:T8)
                    n423 = Unbundle By Name(w550) -> ("RP-IP 2"=w548:string)
                    n424 = Unbundle By Name(w547) -> ("PUMP"=w542:dbl[], "PROBE"=w545:dbl[])
                    n425 = local read "PUMP"() -> (w543:dbl)
                    n426 = local read "PROBE"() -> (w546:dbl)
                    n427 = call "RP-VOA CONVERSION P to V.vi"("Calibration points"=w542, "% power"=w543) -> ("DAC Voltage"=w541:dbl)
                    n428 = call "RP-VOA CONVERSION P to V.vi"("Calibration points"=w545, "% power"=w546) -> ("DAC Voltage"=w544:dbl)
                    n429 = call "RP-ANALOG-OUT.vi"("Voltage"=w544, "Pin #"=w551, "IP address"=w548) -> ()  [unwired: 1 out]
                    n430 = call "RP-ANALOG-OUT.vi"("Voltage"=w541, "Pin #"=w549, "IP address"=w548) -> ()  [unwired: 1 out]
                  }
                  frame #1 {
                    n431 = local read "VNA SETTING CLUSTER"() -> (w555:T4)
                    n432 = local read "PROBE"() -> (w553:dbl)
                    n433 = local read "PUMP"() -> (w554:dbl)
                    n434 = Bundle By Name(cluster=w555, "PUMP"=w554, "PROBE"=w553) -> (w552:T4)
                    n435 = local write "VNA SETTING CLUSTER"(w552) -> ()
                  }
                  frame #2 {
                    n436 = local read "CHANNELS PARAMETERS"() -> (w561:T4[])
                    n437 = local read "CHANNEL CHOICE VNA"() -> (w560:T3)
                    n438 = Index Array(array=w561, index=w560) -> (element=w559:T4)
                    n439 = local read "VNA SETTING CLUSTER"() -> (w558:T4)
                    n440 = Unbundle By Name(w559) -> ("CHANNEL TRACK ?"=w557:bool)
                    n441 = Bundle By Name(cluster=w558, "CHANNEL TRACK ?"=w557) -> (w556:T4)
                    n442 = Replace Array Subset(array=w561, new element=w556, index=w560) -> (w562:T4[])
                    n443 = local write "CHANNELS PARAMETERS"(w562) -> ()
                  }
                }
              }
              frame "SAVE VNA" {
                n444 = local read "TRACK DATA PARAMETERS"() -> (w570:cluster{"MAIN FOLDER":path})
                n445 = Unbundle By Name(w570) -> ("MAIN FOLDER"=w566:path)
                n446 = Build Path(base path=w566, name or relative path=path "SAVED VNA SPECTRUMS ") -> (appended path=w567:path)
                n447 = call <vilib>:"Check if File or Folder Exists.vi"("path"=w567) -> ("file or folder exists?"=w569:bool, "dup path"=w568:path)  [unwired: 8 in, 1 out]
                n448 = case shown="True" w569 {
                  tunnel: [w575 w576] -> w564
                  tunnel: w568 -> [w574 w576]
                  frame False {
                    n449 = Create Folder(path (use dialog)=w574) -> (created path=w575:path)  [unwired: 2 in, 2 out]
                  }
                  frame True {
                  }
                }
                n450 = call "File Dialog"("start path"=w564) -> ("selected path"=w571:path, "cancelled"=w572:bool, "error out"=w563:errorcluster)  [unwired: 11 in, 1 out]
                n451 = case shown="False" w572 {
                  tunnel: w571 -> [w581 _]
                  tunnel: w563 -> [_ _]
                  frame False {
                    n452 = Path To String(path=w581) -> (string=w582:string)
                    n453 = local read "VNA DATA CLUSTER"() -> (w593:T9)
                    n454 = xnode "Match Regular Expression"("input string"=w582, "regular expression"=".txt$") -> ("before match"=w578:string)  [unwired: 4 in, 4 out]
                    n455 = Concatenate Strings(w578, ".txt" ("string")) -> (w577:string)
                    n456 = Unbundle By Name(w593) -> ("FREQUENCY TABLE"=w592:ext[], "MAGNITUDE TABLE"=w591:ext[], "PHASE TABLE"=w590:ext[], "REAL TABLE"=w585:ext[], "IMAGINARY TABLE"=w584:ext[])
                    n457 = String To Path(string=w577) -> (path=w580:path)
                    n458 = Build Array(w592, w591, w590, w585, w584) -> (w588:ext[][])
                    n459 = call-poly <vilib>:"Write Delimited Spreadsheet.vi"("file path (dialog if empty)"=w580, "format (%.3f)"="%.6f", "2D data"=w588, "append to file? (new file:F)"=FALSE, "transpose? (no:F)"=TRUE) -> ()  [unwired: 9 in, 2 out]
                  }
                  frame True {
                  }
                }
              }
              frame "STOP" {
                w713 = FALSE ("TRACK-STOP")
                n460 = local write "STATUS"(w712) -> ()
                n461 = local read "RP CONNECT"() -> (w711:bool)
                n462 = case shown="True" w711 {
                  tunnel: w715 -> [_ w718]
                  tunnel: w714 -> [_ w717]
                  frame False {
                  }
                  frame True {
                    n463 = TCP Close Connection(connection ID=w718, error in (no error)=w717) -> ()  [unwired: 1 in, 2 out]
                  }
                }
                n464 = local write "TRACK-STOP"(w713) -> ()
                n465 = local write "LOOP ACT"(w713) -> ()
              }
            }
          }
          frame Error {
          }
        }
      }
      n466 = while {
        shift-right: [w723] -> w81
        shift-left: w82 -> [w725]
        tunnel: w79 -> [w726]
        tunnel: [w721] -> w72
        stop <- w721 stop-if-true
        n467 = event shown="[4] \"MAGNITUDE/PHASE\": Value Change" {
          selector: _ -> [_ _ _ _ _ _ _ _ _ _ _ _ _ _ _ _ _ _ _ _ _ _ _ _ _ _ _]
          dyn-events: _ -> [_ _ _ _ _ _ _ _ _ _ _ _ _ _ _ _ _ _ _ _ _ _ _ _ _ _ _]
          timeout: 250 -> [_ _ _ _ _ _ _ _ _ _ _ _ _ _ _ _ _ _ _ _ _ _ _ _ _ _ _]
          tunnel: w726 -> [w731 w734 w738 _ _ w770 _ w795 w817 w821 w847 w873 w896 w908 w937 _ _ _ _ _ w950 _ w976 _ w984 _ _]
          tunnel: w725 -> [w729 w733 w737 _ _ w769 _ w794 w816 w820 w846 w875 w895 w907 w936 _ _ _ _ _ w949 _ w977 _ w983 _ _]
          tunnel: [w728 w732 w736 _ _ w768 _ w793 w815 w819 w844 w874 w894 w906 w938 _ _ _ _ _ w948 _ w975 _ w982 _ _] -> w723
          tunnel: [_ _ _ _ _ _ _ _ _ _ _ _ _ _ w934 _ _ _ _ _ _ _ _ _ _ _ _] -> w724
          event "BTN LOOP VNA": Value Change {
            n468 = event-data() -> ("NewVal"=w727:bool)  [unwired: 1 in]
            n469 = local write "LOOP ACT"(w727) -> ()
            n470 = Enqueue Element(queue=w731, element="VNA LOOP", error in (no error)=w729) -> (error out=w728:errorcluster)  [unwired: 1 in, 2 out]
          }
          event "BTN RUN VNA": Mouse Up {
            n471 = event-data() -> ()  [unwired: 1 in, 2 out]
            n472 = Enqueue Element(queue=w734, element="RUN VNA", error in (no error)=w733) -> (error out=w732:errorcluster)  [unwired: 1 in, 2 out]
          }
          event "PUMP", "PROBE": Mouse Up {
            n473 = event-data() -> ()  [unwired: 1 in, 2 out]
            n474 = Enqueue Element(queue=w738, element="POWER UPDATE", error in (no error)=w737) -> (error out=w736:errorcluster)  [unwired: 1 in, 2 out]
          }
          event "Hide/Show track data channel": Value Change {
            # "TO TEST ON ALPHA"
            n475 = event-data() -> ()  [unwired: 1 in, 2 out]
            n476 = local read "Hide/Show track data channel"() -> (w740:bool[])
            n477 = for {
              tunnel: w740 -> [w741] mode=indexing
              i -> [w742]
              n478 = flat-sequence {
                tunnel: w742 -> [w743]
                tunnel: w741 -> [w744]
                frame #0 {
                  n479 = property on="LIVE TRACK" class="WFGraph (strict)"("Active Plot"=w743) -> ()  [unwired: 2 in, 2 out]
                }
                frame #1 {
                  n480 = property on="LIVE TRACK" class="WFGraph (strict)"("Plot.Visible?"=w744) -> ()  [unwired: 2 in, 2 out]
                }
              }
            }
          }
          event "MAGNITUDE/PHASE": Value Change {
            n481 = event-data() -> ()  [unwired: 1 in, 2 out]
            n482 = local read "BTN AUTOSCALE"() -> (w749:bool)
            n483 = case shown="True" w749 {
              frame False {
              }
              frame True {
                n484 = flat-sequence {
                  frame #0 {
                    n485 = property on="MAGNITUDE/PHASE" class="XYGraph (strict)"("ActYScl"=0 ("Active Y Scale")) -> ()  [unwired: 2 in, 2 out]
                  }
                  frame #1 {
                    n486 = local read "BTN DISPLAY TYPE"() -> (w751:bool)
                    n487 = case shown="False" w751 {
                      frame False {
                        n488 = local read "PERSISTANCE DATA CLUSTER"() -> (w761:T9)
                        n489 = local read "VNA DATA CLUSTER"() -> (w765:T9)
                        n490 = local read "BTN VIEW PERSISTANCE"() -> (w758:bool)
                        n491 = Unbundle By Name(w761) -> ("MAGNITUDE TABLE"=w762:ext[])
                        n492 = Unbundle By Name(w765) -> ("MAGNITUDE TABLE"=w766:ext[])
                        n493 = Array Max & Min(array=w762) -> (max value=w756:ext)  [unwired: 3 out]
                        n494 = Array Max & Min(array=w766) -> (max value=w760:ext)  [unwired: 3 out]
                        n495 = Select(t=w756, s=w758, f=0.0 ("t")) -> (s? t:f=w757:ext)
                        n496 = Max & Min(x=w760, y=w757) -> (max(x,y)=w759:ext)  [unwired: 1 out]
                        n497 = Multiply(x=1.1, y=w759) -> (x*y=w754:ext)
                        n498 = Max & Min(x=w754, y=ext 1.0) -> (max(x,y)=w752:ext)  [unwired: 1 out]
                        n499 = property on="MAGNITUDE/PHASE" class="XYGraph (strict)"("YScale.Maximum"=w752, "YScale.Minimum"=0.0) -> ()  [unwired: 2 in, 2 out]
                      }
                      frame True {
                        n500 = property on="MAGNITUDE/PHASE" class="XYGraph (strict)"("YScale.ScaleFit"=u8 1 ("Y Scale.Scale Fit")) -> ()  [unwired: 2 in, 2 out]
                      }
                    }
                  }
                }
              }
            }
            n501 = local read "BTN DISPLAY TYPE"() -> (w746:bool)
            n502 = Select(t="I/Q", s=w746, f="MAGNITUDE/PHASE") -> (s? t:f=w745:string)
            n503 = property on="MAGNITUDE/PHASE" class="XYGraph (strict)"("Caption.Text"=w745) -> ()  [unwired: 2 in, 2 out]
          }
          event "CHANNEL CHOICE VNA": Value Change {
            n504 = event-data() -> ()  [unwired: 1 in, 2 out]
            n505 = Enqueue Element(queue=w770, element="CHANNEL CHANGE", error in (no error)=w769) -> (error out=w768:errorcluster)  [unwired: 1 in, 2 out]
          }
          event "BTN NEW TRACK": Mouse Up {
            n506 = event-data() -> ()  [unwired: 1 in, 2 out]
            n507 = Two Button Dialog(message="Initiate a new tracking session ?") -> (T button?=w772:bool)  [unwired: 2 in]
            n508 = case shown="True" w772 {
              frame False {
              }
              frame True {
                n509 = stacked-sequence {
                  frame #0 {
                    # "LOCK ALL CONTROLS"
                  }
                  frame #1 {
                    n510 = local read "ASSAY NAME"() -> (w779:string)
                    n511 = local read "CHANNELS PARAMETERS"() -> (w780:T4[])
                    n512 = local read "TRACK DATA PARAMETERS"() -> (w778:cluster{"MAIN FOLDER":path})
                    n513 = Unbundle By Name(w778) -> ("MAIN FOLDER"=w777:path)
                    n514 = call "RP-TRACKDataStructBuild.vi"("CHANNELS PARAMETERS"=w780, "Track session name"=w779, "SensWay track data path"=w777) -> ("TRACK REPOSITERY"=w776:path, "Track File List"=w775:path[], "Track Repositery List"=w774:path[])
                    n515 = local write "Track Repositery List"(w774) -> ()
                    n516 = local write "Track File List"(w775) -> ()
                    n517 = local write "TRACK REPOSITERY"(w776) -> ()
                  }
                  frame #2 {
                    n518 = local read "CHANNELS PARAMETERS"() -> (w782:T4[])
                    n519 = for {
                      tunnel: w782 -> [w792] mode=indexing
                      border: cluster{"CHANNEL":dbl, "KPI 1 TRACK":ext[]}[] [] -> [_]
                      i -> [w788]
                      n520 = Unbundle By Name(w792) -> ("CHANNEL TRACK ?"=w783:bool)
                      n521 = Select(t=dbl[] [0.0], s=w783, f=dbl[] []) -> (s? t:f=w786:dbl[])
                      n522 = Bundle By Name(cluster=cluster{"CHANNEL":dbl, "KPI 1 TRACK":ext[]} {"CHANNEL"=0.0, "KPI 1 TRACK"=[0.0]} ("TRACK DATA CLUSTER"), "CHANNEL"=w788, "KPI 1 TRACK"=w786) -> (w787:cluster{"CHANNEL":dbl, "KPI 1 TRACK":ext[]})
                      n523 = feedback #1() -> (w790:cluster{"CHANNEL":dbl, "KPI 1 TRACK":ext[]}[])
                      n524 = Build Array (concatenate)(w790, w787) -> (w791:cluster{"CHANNEL":dbl, "KPI 1 TRACK":ext[]}[])
                      n525 = feedback-in #1(w791) -> ()
                      n526 = local write "TRACK DATA CLUSTER TBL"(w791) -> ()
                    }
                  }
                  frame #3 {
                  }
                }
              }
            }
          }
          event "START", "STOP": Value Change {
            n527 = event-data() -> ()  [unwired: 1 in, 1 out]
            n528 = stacked-sequence {
              frame #0 {
                n529 = local read "STOP"() -> (w801:dbl)
                n530 = local read "START"() -> (w800:dbl)
                n531 = Subtract(x=w801, y=w800) -> (x-y=w802:dbl)
                n532 = Add(x=w801, y=w800) -> (x+y=w799:dbl)
                n533 = local write "SPAN"(w802) -> ()
                n534 = Divide(x=w799, y=2.0) -> (x/y=w797:dbl)
                n535 = local write "CENTER"(w797) -> ()
              }
              frame #1 {
                n536 = local read "Points N°"() -> (w807:i32)
                n537 = local read "SPAN"() -> (w806:dbl)
                n538 = Divide(x=w806, y=w807) -> (x/y=w805:dbl)
                n539 = Multiply(x=w805, y=1000.0) -> (x*y=w804:dbl)
                n540 = local write "SPACING"(w804) -> ()
              }
              frame #2 {
                w808 = 1000
                n541 = local read "STOP"() -> (w810:dbl)
                n542 = local read "START"() -> (w812:dbl)
                n543 = Multiply(x=w812, y=w808) -> (x*y=w811:dbl)
                n544 = Multiply(x=w808, y=w810) -> (x*y=w809:dbl)
                n545 = local read "RP VNA SETTING"() -> (w814:T1)
                n546 = Bundle By Name(cluster=w814, "F start"=w811, "F stop"=w809) -> (w813:T1)
                n547 = local write "RP VNA SETTING"(w813) -> ()
              }
            }
            n548 = Enqueue Element(queue=w795, element="UPDATE", error in (no error)=w794) -> (error out=w793:errorcluster)  [unwired: 1 in, 2 out]
          }
          event "AVG Nb", "BTN AVG ENABLE": Value Change {
            n549 = event-data() -> ()  [unwired: 1 in, 1 out]
            n550 = Enqueue Element(queue=w817, element="UPDATE", error in (no error)=w816) -> (error out=w815:errorcluster)  [unwired: 1 in, 2 out]
          }
          event "CENTER", "SPAN": Value Change {
            n551 = event-data() -> ()  [unwired: 1 in, 1 out]
            n552 = stacked-sequence {
              frame #0 {
                w824 = 100.0 ("y")
                n553 = local read "CENTER"() -> (w828:dbl)
                n554 = local read "SPAN"() -> (w830:dbl)
                n555 = Divide(x=w830, y=2.0) -> (x/y=w827:dbl)
                n556 = Subtract(x=w828, y=w827) -> (x-y=w825:dbl)
                n557 = Add(x=w828, y=w827) -> (x+y=w831:dbl)
                n558 = local write "STOP"(w831) -> ()
                n559 = Greater Or Equal?(x=w825, y=w824) -> (x >= y?=w826:bool)
                n560 = Select(t=w825, s=w826, f=w824) -> (s? t:f=w823:dbl)
                n561 = local write "START"(w823) -> ()
              }
              frame #1 {
                n562 = local read "Points N°"() -> (w836:i32)
                n563 = local read "SPAN"() -> (w835:dbl)
                n564 = Divide(x=w835, y=w836) -> (x/y=w834:dbl)
                n565 = Multiply(x=w834, y=1000.0) -> (x*y=w833:dbl)
                n566 = local write "SPACING"(w833) -> ()
              }
              frame #2 {
                w837 = 1000
                n567 = local read "STOP"() -> (w839:dbl)
                n568 = local read "START"() -> (w841:dbl)
                n569 = Multiply(x=w841, y=w837) -> (x*y=w840:dbl)
                n570 = Multiply(x=w837, y=w839) -> (x*y=w838:dbl)
                n571 = local read "RP VNA SETTING"() -> (w843:T1)
                n572 = Bundle By Name(cluster=w843, "F start"=w840, "F stop"=w838) -> (w842:T1)
                n573 = local write "RP VNA SETTING"(w842) -> ()
              }
            }
            n574 = Enqueue Element(queue=w821, element="UPDATE", error in (no error)=w820) -> (error out=w819:errorcluster)  [unwired: 1 in, 2 out]
          }
          event "BTN ZOOM+": Mouse Up; "BTN ZOOM+": Value Change {
            n575 = event-data() -> ()  [unwired: 1 in, 1 out]
            n576 = stacked-sequence {
              frame #0 {
                n577 = local read "SPAN"() -> (w850:dbl)
                n578 = Multiply(x=w850, y=0.8) -> (x*y=w848:dbl)
                n579 = local write "SPAN"(w848) -> ()
              }
              frame #1 {
                n580 = local read "Points N°"() -> (w855:i32)
                n581 = local read "SPAN"() -> (w854:dbl)
                n582 = Divide(x=w854, y=w855) -> (x/y=w853:dbl)
                n583 = Multiply(x=w853, y=1000.0) -> (x*y=w852:dbl)
                n584 = local write "SPACING"(w852) -> ()
              }
              frame #2 {
                w857 = 100.0 ("y")
                n585 = local read "SPAN"() -> (w860:dbl)
                n586 = local read "CENTER"() -> (w862:dbl)
                n587 = Divide(x=w860, y=2.0) -> (x/y=w861:dbl)
                n588 = Subtract(x=w862, y=w861) -> (x-y=w858:dbl)
                n589 = Add(x=w862, y=w861) -> (x+y=w864:dbl)
                n590 = local write "STOP"(w864) -> ()
                n591 = Greater Or Equal?(x=w858, y=w857) -> (x >= y?=w859:bool)
                n592 = Select(t=w858, s=w859, f=w857) -> (s? t:f=w856:dbl)
                n593 = local write "START"(w856) -> ()
              }
              frame #3 {
                w865 = 1000
                n594 = local read "STOP"() -> (w867:dbl)
                n595 = local read "START"() -> (w869:dbl)
                n596 = Multiply(x=w869, y=w865) -> (x*y=w868:dbl)
                n597 = Multiply(x=w865, y=w867) -> (x*y=w866:dbl)
                n598 = local read "RP VNA SETTING"() -> (w871:T1)
                n599 = Bundle By Name(cluster=w871, "F start"=w868, "F stop"=w866) -> (w870:T1)
                n600 = local write "RP VNA SETTING"(w870) -> ()
              }
            }
            n601 = Enqueue Element(queue=w847, element="UPDATE", error in (no error)=w846) -> (error out=w844:errorcluster)  [unwired: 1 in, 2 out]
          }
          event "BTN RESET VNA": Mouse Up {
            n602 = event-data() -> ()  [unwired: 1 in, 1 out]
            n603 = flat-sequence {
              tunnel: w873 -> [w877]
              tunnel: [w877] -> w872
              frame #0 {
                w886 = u32 1000 ("Decimation")
                w884 = u32 2000000 ("Decimation")
                w885 = u32 200000 ("Decimation")
                w879 = u32 32700 ("F_corr")
                n604 = local read "RP VNA SETTING"() -> (w889:T1)
                n605 = local read "Points N°"() -> (w887:i32)
                n606 = Bundle By Name(cluster=w889, "F start"=w885, "F stop"=w884, "Sweep size"=w887, "Decimation"=u32 5000, "F_corr"=u32 0, "Ph_OUT1"=u32 0, "Ph_OUT2"=u32 0 ("F_corr"), "OUT_Lvl1"=w879, "OUT_Lvl2"=w879, "GPIO"=u32 0 ("F_corr")) -> (w888:T1)
                n607 = local write "RP VNA SETTING"(w888) -> ()
                n608 = Divide(x=w884, y=w886) -> (x/y=w890:dbl)
                n609 = Divide(x=w885, y=w886) -> (x/y=w891:dbl)
                n610 = local write "CENTER"(1050.0 ("Center")) -> ()
                n611 = local write "SPAN"(1900.0 ("Center")) -> ()
                n612 = local write "START"(w891) -> ()
                n613 = local write "STOP"(w890) -> ()
              }
            }
            n614 = Enqueue Element(queue=w872, element="UPDATE", error in (no error)=w875) -> (error out=w874:errorcluster)  [unwired: 1 in, 2 out]
          }
          event "Points N°": Value Change {
            n615 = event-data() -> ()  [unwired: 1 in, 1 out]
            n616 = stacked-sequence {
              frame #0 {
                n617 = local read "Points N°"() -> (w902:i32)
                n618 = local read "SPAN"() -> (w901:dbl)
                n619 = Divide(x=w901, y=w902) -> (x/y=w900:dbl)
                n620 = Multiply(x=w900, y=1000.0) -> (x*y=w899:dbl)
                n621 = local write "SPACING"(w899) -> ()
              }
              frame #1 {
                n622 = local read "Points N°"() -> (w903:i32)
                n623 = local read "RP VNA SETTING"() -> (w905:T1)
                n624 = Bundle By Name(cluster=w905, "Sweep size"=w903) -> (w904:T1)
                n625 = local write "RP VNA SETTING"(w904) -> ()
              }
            }
            n626 = Enqueue Element(queue=w896, element="UPDATE", error in (no error)=w895) -> (error out=w894:errorcluster)  [unwired: 1 in, 2 out]
          }
          event "BTN ZOOM-": Mouse Up {
            n627 = event-data() -> ()  [unwired: 1 in, 1 out]
            n628 = stacked-sequence {
              frame #0 {
                n629 = local read "SPAN"() -> (w912:dbl)
                n630 = Multiply(x=w912, y=1.2) -> (x*y=w910:dbl)
                n631 = local write "SPAN"(w910) -> ()
              }
              frame #1 {
                n632 = local read "Points N°"() -> (w917:i32)
                n633 = local read "SPAN"() -> (w916:dbl)
                n634 = Divide(x=w916, y=w917) -> (x/y=w915:dbl)
                n635 = Multiply(x=w915, y=1000.0) -> (x*y=w914:dbl)
                n636 = local write "SPACING"(w914) -> ()
              }
              frame #2 {
                w920 = 100.0 ("y")
                n637 = local read "SPAN"() -> (w922:dbl)
                n638 = local read "CENTER"() -> (w925:dbl)
                n639 = Divide(x=w922, y=2.0) -> (x/y=w924:dbl)
                n640 = Subtract(x=w925, y=w924) -> (x-y=w918:dbl)
                n641 = Add(x=w925, y=w924) -> (x+y=w926:dbl)
                n642 = Greater Or Equal?(x=w918, y=w920) -> (x >= y?=w921:bool)
                n643 = Select(t=w918, s=w921, f=w920) -> (s? t:f=w919:dbl)
                n644 = local write "STOP"(w926) -> ()
                n645 = local write "START"(w919) -> ()
              }
              frame #3 {
                w927 = 1000
                n646 = local read "STOP"() -> (w929:dbl)
                n647 = local read "START"() -> (w931:dbl)
                n648 = Multiply(x=w931, y=w927) -> (x*y=w930:dbl)
                n649 = Multiply(x=w927, y=w929) -> (x*y=w928:dbl)
                n650 = local read "RP VNA SETTING"() -> (w933:T1)
                n651 = Bundle By Name(cluster=w933, "F start"=w930, "F stop"=w928) -> (w932:T1)
                n652 = local write "RP VNA SETTING"(w932) -> ()
              }
            }
            n653 = Enqueue Element(queue=w908, element="UPDATE", error in (no error)=w907) -> (error out=w906:errorcluster)  [unwired: 1 in, 2 out]
          }
          event "BTN STOP": Value Change {
            n654 = event-data() -> ()  [unwired: 1 in, 1 out]
            n655 = Two Button Dialog(message="Are you sure you want to exit ?") -> (T button?=w934:bool)  [unwired: 2 in]
            n656 = case shown="True" w934 {
              tunnel: [w939 w942] -> w938
              tunnel: w937 -> [_ w941]
              tunnel: w936 -> [w939 w940]
              frame False {
              }
              frame True {
                n657 = Enqueue Element(queue=w941, element="STOP", error in (no error)=w940) -> (error out=w942:errorcluster)  [unwired: 1 in, 2 out]
              }
            }
          }
          event "PANEL GENERAL SETTINGS": Value Change {
            n658 = event-data() -> ()  [unwired: 1 in, 2 out]
            n659 = local write "MAIN TAB"(enum32{"Page 1", "Page 4", "Page 2", "Page 3"}."Page 3" ("Tab Control")) -> ()
          }
          event Timeout {
            n660 = event-data() -> ()  [unwired: 1 in, 2 out]
          }
          event "PANEL TRACK SETTINGS": Value Change {
            n661 = event-data() -> ()  [unwired: 1 in, 2 out]
            n662 = local write "MAIN TAB"(enum32{"Page 1", "Page 4", "Page 2", "Page 3"}."Page 2" ("Tab Control")) -> ()
          }
          event "PANEL VNA": Value Change {
            n663 = event-data() -> ()  [unwired: 1 in, 2 out]
            n664 = local write "MAIN TAB"(enum32{"Page 1", "Page 4", "Page 2", "Page 3"}."Page 1" ("Tab Control")) -> ()
          }
          event "PANEL TRACKING": Value Change {
            n665 = event-data() -> ()  [unwired: 1 in, 2 out]
            n666 = local write "MAIN TAB"(enum32{"Page 1", "Page 4", "Page 2", "Page 3"}."Page 4" ("Tab Control")) -> ()
          }
          event "BTN Center to max": Mouse Up; "BTN Center to max": Value Change {
            n667 = event-data() -> ()  [unwired: 1 in, 2 out]
            n668 = stacked-sequence {
              frame #0 {
                # "ATTENTION ! CONFUSION  freq table"
                n669 = local read "VNA DATA CLUSTER"() -> (w955:T9)
                n670 = Unbundle By Name(w955) -> ("FREQUENCY TABLE"=w954:ext[], "MAGNITUDE TABLE"=w953:ext[])
                n671 = Array Max & Min(array=w953) -> (max index (indices)=w958:i32)  [unwired: 3 out]
                n672 = Index Array(array=w954, index=w958) -> (element=w957:ext)
                n673 = Divide(x=w957, y=1000.0) -> (x/y=w952:ext)
                n674 = local write "CENTER"(w952) -> ()
                n675 = property on="CENTER" class="DigNum (strict)"("Val(Sgnl)"=w952) -> ()  [unwired: 2 in, 2 out]
              }
              frame #1 {
                w961 = 1000
                n676 = local read "START"() -> (w959:dbl)
                n677 = local read "STOP"() -> (w960:dbl)
                n678 = Multiply(x=w959, y=w961) -> (x*y=w963:dbl)
                n679 = Multiply(x=w961, y=w960) -> (x*y=w962:dbl)
                n680 = local read "RP VNA SETTING"() -> (w965:T1)
                n681 = Bundle By Name(cluster=w965, "F start"=w963, "F stop"=w962) -> (w964:T1)
                n682 = local write "RP VNA SETTING"(w964) -> ()
              }
            }
            n683 = Enqueue Element(queue=w950, element="UPDATE", error in (no error)=w949) -> (error out=w948:errorcluster)  [unwired: 1 in, 2 out]
          }
          event "BTN AF VNA": Mouse Up {
            n684 = event-data() -> ()  [unwired: 1 in, 2 out]
            n685 = local read "AUTOFOCUS PARAMETERS"() -> (w967:cluster{"ITERATIONS":i32})
            n686 = Unbundle By Name(w967) -> ("ITERATIONS"=w966:i32)
            n687 = for {
              N: w966 -> [_]
              tunnel: [w970] -> w968
              n688 = flat-sequence {
                tunnel: [w971] -> w970
                frame #0 {
                  w971 = FALSE ("Valeur (Signalisation)")
                  n689 = property on="BTN Center to max" class="Bool (strict)"("Val(Sgnl)"=w971) -> ()  [unwired: 2 in, 2 out]
                }
                frame #1 {
                  n690 = property on="BTN ZOOM+" class="Bool (strict)"("Val(Sgnl)"=FALSE ("Valeur (Signalisation)")) -> ()  [unwired: 2 in, 2 out]
                }
              }
              n691 = Wait (ms)(milliseconds to wait=u32 250 ("attente (ms)")) -> ()  [unwired: 1 out]
            }
            n692 = property on="BTN Center to max" class="Bool (strict)"("Val(Sgnl)"=w968) -> ()  [unwired: 2 in, 2 out]
          }
          event "BTN RUN TRACK": Value Change {
            w973 = TRUE ("x")
            n693 = event-data() -> ()  [unwired: 1 in, 2 out]
            n694 = Not(x=w973) -> (.not. x?=w974:bool)
            n695 = local write "LOOP ACT"(w973) -> ()
            n696 = property on="BTN PAUSE TRACK" class="Bool (strict)"("Visible"=w973) -> ()  [unwired: 2 in, 2 out]
            n697 = Enqueue Element(queue=w976, element="TRACK", error in (no error)=w977) -> (error out=w975:errorcluster)  [unwired: 1 in, 2 out]
            n698 = property on="BTN RUN TRACK" class="Bool (strict)"("Visible"=w974) -> ()  [unwired: 2 in, 2 out]
          }
          event "BTN PAUSE TRACK": Mouse Up {
            w979 = FALSE ("x")
            n699 = event-data() -> ()  [unwired: 1 in, 2 out]
            n700 = Not(x=w979) -> (.not. x?=w980:bool)
            n701 = local write "LOOP ACT"(w979) -> ()
            n702 = property on="BTN PAUSE TRACK" class="Bool (strict)"("Visible"=w979) -> ()  [unwired: 2 in, 2 out]
            n703 = property on="BTN RUN TRACK" class="Bool (strict)"("Visible"=w980) -> ()  [unwired: 2 in, 2 out]
          }
          event "BTN SAVE VNA": Mouse Up {
            n704 = event-data() -> ()  [unwired: 1 in, 2 out]
            n705 = Enqueue Element(queue=w984, element="SAVE VNA", error in (no error)=w983) -> (error out=w982:errorcluster)  [unwired: 1 in, 2 out]
          }
          event "BTN VIEW PERSISTANCE": Value Change {
            n706 = event-data() -> ("NewVal"=w985:bool)  [unwired: 1 in, 1 out]
            n707 = case shown="True" w985 {
              frame False {
              }
              frame True {
                n708 = local read "VNA DATA CLUSTER"() -> (w986:T9)
                n709 = local write "PERSISTANCE DATA CLUSTER"(w986) -> ()
              }
            }
          }
          event "BTN DISPLAY TYPE": Value Change {
            n710 = event-data() -> ("NewVal"=w987:bool)  [unwired: 1 in, 1 out]
            n711 = case shown="True" w987 {
              frame False {
                n712 = property on="BTN FIT DISPLAY" class="Bool (strict)"("DisabledEnum"=T11."Enabled" ("Disabled")) -> ()  [unwired: 2 in, 2 out]
              }
              frame True {
                n713 = property on="BTN FIT DISPLAY" class="Bool (strict)"("DisabledEnum"=T11."Disabled and Grayed Out" ("Disabled"), "Value"=FALSE ("Fit display")) -> ()  [unwired: 2 in, 2 out]
              }
            }
          }
        }
        n714 = Or(x=w723, y=w724) -> (x .or. y?=w721:bool)
        n715 = Wait (ms)(milliseconds to wait=u32 50 ("attente (ms)")) -> ()  [unwired: 1 out]
      }
      n716 = And(x=w72, y=w71) -> (x .and. y?=w70:bool)
      n717 = case shown="True" w70 {
        tunnel: w81 -> [_ w85]
        tunnel: w79 -> [_ w84]
        frame False {
        }
        frame True {
          n718 = Release Queue(queue=w84, error in (no error)=w85) -> ()  [unwired: 1 in, 3 out]
          n719 = property on="MAIN TAB" class="TabCtl (strict)"("Tabs Visible?"=TRUE ("Onglets visibles ?")) -> ()  [unwired: 2 in, 2 out]
        }
      }
    }
  }
